vi "ParameterAnalyzer Loop.vi"(6 "Used functions":bool, 8 "error in":errorcluster, 9 "IBM OptoElectroMechanics Configuration":T1={"Parameter Analizer"={"Parameter Analyzer VISA Session"="COM1", "Sweeping Time Parameters"={"Integration Time"=0, "Short Integration Time (s)"=1.0, "Long Integration Time (s)"=0.0, "Wait Time Parameter"=1.0}, "Acquisition Mode"=enum."Sweeping Mode", "Status Polling Time (ms)"=0, "Comment"="Test VI", "SMU 1 - Sweeping"={"Start / Offset"=0.0, "Stop / Ratio"=1.0, "Step \n(linear only)"=0.01, "Compliance"=0.1, "Power \nCompliance"=0.0, "Mode"=0, "Function"=0, "Sweep Mode"=FALSE}, "SMU 2 - Sweeping"={"Start / Offset"=0.0, "Stop / Ratio"=1.0, "Step \n(linear only)"=0.01, "Compliance"=0.1, "Power \nCompliance"=0.0, "Mode"=0, "Function"=0, "Sweep Mode"=FALSE}, "SMU 3 - Sweeping"={"Start / Offset"=0.0, "Stop / Ratio"=1.0, "Step \n(linear only)"=0.01, "Compliance"=0.1, "Power \nCompliance"=0.0, "Mode"=0, "Function"=0, "Sweep Mode"=FALSE}, "SMU 4 - Sweeping"={"Start / Offset"=0.0, "Stop / Ratio"=1.0, "Step \n(linear only)"=0.01, "Compliance"=0.1, "Power \nCompliance"=0.0, "Mode"=0, "Function"=0, "Sweep Mode"=FALSE}, "Sweep Spacing"=0, "Range"=0, "SMU1 - Sampling"={"Source"=10.0, "Compliance"=1e-05, "Mode"=0, "Function"=FALSE}, "SMU2 - Sampling"={"Source"=1.0, "Compliance"=1.0, "Mode"=0, "Function"=FALSE}, "SMU3 - Sampling"={"Source"=10.0, "Compliance"=1e-05, "Mode"=0, "Function"=FALSE}, "SMU4 - Sampling"={"Source"=0.1, "Compliance"=60.0, "Mode"=10, "Function"=FALSE}, "Sampling Time Parameters"={"Initial Interval (s)"=0.1, "Number of Samples"=60, "Total Sampling Time (s)"=10.0, "Hold Time (s)"=0.0, "Sampling Mode"=0, "Sampling Time"=0}, "Stop Condition"={"Enable Delay (s)"=0.0, "Name"="", "Threshold"=0.0, "num. of events"=1, "Event"=0, "Stop Condition Enable"=FALSE}}, "Switching Matrix"={"Switching Matrix VISA Session"="GPIB0::18::INSTR", "Connections"=[{"Connections"=[FALSE, FALSE, FALSE, FALSE, FALSE, FALSE, FALSE, FALSE, FALSE, FALSE, FALSE, FALSE], "Connection Type"=enum."Disconnected"}, {"Connections"=[FALSE, FALSE, FALSE, FALSE, FALSE, FALSE, FALSE, FALSE, FALSE, FALSE, FALSE, FALSE], "Connection Type"=enum."Disconnected"}, {"Connections"=[FALSE, FALSE, FALSE, FALSE, FALSE, FALSE, FALSE, FALSE, FALSE, FALSE, FALSE, FALSE], "Connection Type"=enum."Disconnected"}, {"Connections"=[FALSE, FALSE, FALSE, FALSE, FALSE, FALSE, FALSE, FALSE, FALSE, FALSE, FALSE, FALSE], "Connection Type"=enum."Disconnected"}, {"Connections"=[FALSE, FALSE, FALSE, FALSE, FALSE, FALSE, FALSE, FALSE, FALSE, FALSE, FALSE, FALSE], "Connection Type"=enum."Disconnected"}, {"Connections"=[FALSE, FALSE, FALSE, FALSE, FALSE, FALSE, FALSE, FALSE, FALSE, FALSE, FALSE, FALSE], "Connection Type"=enum."Disconnected"}, {"Connections"=[FALSE, FALSE, FALSE, FALSE, FALSE, FALSE, FALSE, FALSE, FALSE, FALSE, FALSE, FALSE], "Connection Type"=enum."Disconnected"}, {"Connections"=[FALSE, FALSE, FALSE, FALSE, FALSE, FALSE, FALSE, FALSE, FALSE, FALSE, FALSE, FALSE], "Connection Type"=enum."Disconnected"}]}, "Stress Control"={"Stress Control VISA Session"="StrainMotor", "Axis"=0, "Motion"=0, "Destination (°)"=0.0, "Speed (°/s)"=4.0, "Position (°)"=25.0}, "Optical Spectrometer"={"Laser Settings"={"Laser Wavelength"=enum."365 nm", "Neutral Density Filter"=enum."100%"}, "Spectrometer Settings"={"Confocal Hole Size (µm)"=0.0, "Grating"=2, "Detector"=enum."InGaAs Array"}, "Acquisition Settings"={"Acquisition Mode"=enum."Multi-Window", "Spectal Position (nm)"=632.0, "From (nm)"=735.0, "To (nm)"=0.0, "Integration Time (s)"=0.0, "Number of Accumulations"=3, "AutoScanning"=FALSE, "Spike Removal"=FALSE}, "Path"=path "C:/07 - Prizes and Awards/Marie Curie Prize/Reply Editors Final NCOMMS(10).docx"}, "Switches & Mirrors"={"Relay VISA Session"="COM1", "Switches"={"Laser"=FALSE, "Video"=FALSE}, "Delays (ms)"={"Laser"=500, "Video"=1500}}, "Camera"={"Settings"={"Pixel clock"=20, "Frame rate"=30.0, "Exposure time"=33.21525, "Master Gain"=0, "Red Gain"=0, "Green Gain"=0, "Blue Gain"=0, "Auto Gain"=FALSE, "White-balance"=FALSE, "Color Correction"=FALSE}}, "XYZ Stage"={"Connection Settings"={"Tango VISA"="", "Baudrate"=57600, "Show Protocol?"=FALSE}, "Manual Control"={"North"=FALSE, "South"=FALSE, "West"=FALSE, "East"=FALSE, "Up"=FALSE, "Down"=FALSE, "Stop"=FALSE, "XY Step"=0.0, "Z step"=0.0}, "Coordinate Control"={"Motion Mode"=enum."Absolute", "Destination [mm]"=[]}}, "AutoFocus"={"Matching Criteria"={"Minimum Score"=700.0, "Color Score Weight"=700.0, "Minimum Contrast"=50, "Match Mode"=0, "Match Feature Mode"=0, "Subpixel Accuracy"=TRUE, "Color Sensitivity"=1, "Search Strategy"=1}, "Z Scan Parameters"={"Z Range"=1380.0, "Resolution"=5000.0, "Initial Direction"=enum."Up", "Focus Threshold"=0.1, "Ascent Constant"=0.1}, "Displacement"=0.0, "Transformation Matrix"=[]}, "Sava Data"={"Workspace Info"={"Device Name"="ProberHead_Tst_C29K3_7(2)", "Device Info"="ProberHead_Tst_C29", "Path"=path "C:/Users/gio/Desktop/ProbeHeadTest"}, "Instrument Configuration"={"Instrument"=enum."Unknown Instrument", "Configuration"="Test Configuration"}, "Stress Motor Position"=0.0, "Electrical Measurement"={"Sequence"=[], "V1"=[], "V2"=[], "V3"=[], "V4"=[], "I1"=[], "I2"=[], "I3"=[], "I4"=[]}, "Optical Spectrum"={"Intensity"=[], "Wavelength"=[], "Energy"=[], "Raman Shift"=[], "Detector Temperature"=0.0}}, "PlotData"={"Sliders"={"Strain Sequence"=0, "Instrument Sequence"=0}, "Measurement"={"Which Instrument?"=enum."No Plot", "Electrical Measurement"={"Sequence"=[], "V1"=[], "V2"=[], "V3"=[], "V4"=[], "I1"=[], "I2"=[], "I3"=[], "I4"=[]}, "Measurement Mode"=enum."Sweeping Mode", "Optical Spectrum"={"Intensity"=[], "Wavelength"=[], "Energy"=[], "Raman Shift"=[], "Detector Temperature"=0.0}}, "Instrument Steps"=[], "Strain Points"=[]}, "Instrument Sequence"={"Caller VI"=enum."User"}, "Strain Measurement"={"Stress Sequence "={"Max Motor Position"=1380.0, "# Intermediate Points"=5000, "Initial Direction"=enum."Tension"}, "Track?"=FALSE}} {"AutoFocus"."Displacement" scale=1.0..1000.0; "AutoFocus"."Z Scan Parameters"."Focus Threshold" min=0.0 max=1000.0 step=1.0 format="%#_2f"; "AutoFocus"."Z Scan Parameters"."Ascent Constant" min=0.0 max=1000.0 step=1.0 format="%#_2f"; "AutoFocus"."Z Scan Parameters"."Resolution" min=0.0 max=1.0 step=0.01 format="%_2g"; "AutoFocus"."Z Scan Parameters"."Z Range" format="%_3g"; "AutoFocus"."Matching Criteria"."Match Mode" items=["Shift Invariant", "Rotation Invariant"]; "AutoFocus"."Matching Criteria"."Match Feature Mode" items=["Color and Shape", "Color", "Shape"]; "AutoFocus"."Matching Criteria"."Color Sensitivity" items=["Low Sensitivity", "Medium Sensitivity", "High Sensitivity"]; "AutoFocus"."Matching Criteria"."Search Strategy" items=["Conservative", "Balance", "Aggressive", "Very Aggressive"]; "XYZ Stage"."Manual Control"."Z step" scale=0.1..10.0; "XYZ Stage"."Manual Control"."XY Step" scale=0.1..1000.0; "Camera"."Settings"."Blue Gain" min=0 max=100 scale=0.0..100.0; "Camera"."Settings"."Green Gain" min=0 max=100 scale=0.0..100.0; "Camera"."Settings"."Red Gain" min=0 max=100 scale=0.0..100.0; "Camera"."Settings"."Master Gain" min=0 max=100 scale=0.0..100.0; "Camera"."Settings"."Exposure time" min=0.101625 max=159.246375 step=0.101625 scale=0.101625..159.246375 scale format="%#.3g"; "Camera"."Settings"."Frame rate" min=2.7455631699174137 max=6.2675785993528725 step=0.000101625 scale=2.7455631699174137..6.2675785993528725 scale format="%^#_3g"; "Camera"."Settings"."Pixel clock" min=5 max=43 scale=5.0..43.0; "PlotData"."Sliders"."Instrument Sequence" scale=0.0..10.0; "PlotData"."Sliders"."Strain Sequence" scale=0.0..10.0; "Strain Measurement"."Stress Sequence"."# Intermediate Points" max=1390; "Parameter Analizer"."Stop Condition"."Event" items=["Value > Threshold", "Value < Threshold", "| Value | > | Threshold |", "| Value | < | Threshold |"]; "Parameter Analizer"."Stop Condition"."Threshold" format="%^.2e"; "Parameter Analizer"."Stop Condition"."Enable Delay (s)" format="%.1f"; "Parameter Analizer"."Sampling Time Parameters"."Sampling Time" items=["Auto (linear only)", "No Limit", "Set Limit"]; "Parameter Analizer"."Sampling Time Parameters"."Sampling Mode" items=["Linear", "Log10", "Log25", "Log50", "Thinned Out"]; "Parameter Analizer"."Sampling Time Parameters"."Hold Time (s)" format="%.4f"; "Parameter Analizer"."Sampling Time Parameters"."Total Sampling Time (s)" format="%.1f"; "Parameter Analizer"."Sampling Time Parameters"."Initial Interval (s)" format="%^.3e"; "Parameter Analizer"."SMU 4 - Sweeping"."Function" items=["Disabled", "Var 1", "Var 2", "Var 1'", "Constant"]; "Parameter Analizer"."SMU 4 - Sweeping"."Mode" items=["V", "I", "V pulse", "I  pulse", "Common"]; "Parameter Analizer"."SMU 4 - Sweeping"."Power \nCompliance" format="%^.2e"; "Parameter Analizer"."SMU 4 - Sweeping"."Compliance" format="%^.2e"; "Parameter Analizer"."SMU 4 - Sweeping"."Step \n(linear only)" format="%^.4e"; "Parameter Analizer"."SMU 4 - Sweeping"."Stop / Ratio" format="%^.4e"; "Parameter Analizer"."SMU 4 - Sweeping"."Start / Offset" format="%^.4e"; "Parameter Analizer"."SMU 3 - Sweeping"."Function" items=["Disabled", "Var 1", "Var 2", "Var 1'", "Constant"]; "Parameter Analizer"."SMU 3 - Sweeping"."Mode" items=["V", "I", "V pulse", "I  pulse", "Common"]; "Parameter Analizer"."SMU 3 - Sweeping"."Power \nCompliance" format="%^.2e"; "Parameter Analizer"."SMU 3 - Sweeping"."Compliance" format="%^.2e"; "Parameter Analizer"."SMU 3 - Sweeping"."Step \n(linear only)" format="%^.4e"; "Parameter Analizer"."SMU 3 - Sweeping"."Stop / Ratio" format="%^.4e"; "Parameter Analizer"."SMU 3 - Sweeping"."Start / Offset" format="%^.4e"; "Parameter Analizer"."SMU 2 - Sweeping"."Function" items=["Disabled", "Var 1", "Var 2", "Var 1'", "Constant"]; "Parameter Analizer"."SMU 2 - Sweeping"."Mode" items=["V", "I", "V pulse", "I  pulse", "Common"]; "Parameter Analizer"."SMU 2 - Sweeping"."Power \nCompliance" format="%^.2e"; "Parameter Analizer"."SMU 2 - Sweeping"."Compliance" format="%^.2e"; "Parameter Analizer"."SMU 2 - Sweeping"."Step \n(linear only)" format="%^.4e"; "Parameter Analizer"."SMU 2 - Sweeping"."Stop / Ratio" format="%^.4e"; "Parameter Analizer"."SMU 2 - Sweeping"."Start / Offset" format="%^.4e"; "Parameter Analizer"."SMU 1 - Sweeping"."Function" items=["Disabled", "Var 1", "Var 2", "Var 1'", "Constant"]; "Parameter Analizer"."SMU 1 - Sweeping"."Mode" items=["V", "I", "V pulse", "I  pulse", "Common"]; "Parameter Analizer"."SMU 1 - Sweeping"."Power \nCompliance" format="%^.2e"; "Parameter Analizer"."SMU 1 - Sweeping"."Compliance" format="%^.2e"; "Parameter Analizer"."SMU 1 - Sweeping"."Step \n(linear only)" format="%^.4e"; "Parameter Analizer"."SMU 1 - Sweeping"."Stop / Ratio" format="%^.4e"; "Parameter Analizer"."SMU 1 - Sweeping"."Start / Offset" format="%^.4e"; "Parameter Analizer"."Sweeping Time Parameters"."Long Integration Time (s)" scale=0.02..2.0; "Parameter Analizer"."Sweeping Time Parameters"."Short Integration Time (s)" scale=8e-05..0.00192; "Parameter Analizer"."Sweeping Time Parameters"."Integration Time" items=["Short", "Long"]; "Parameter Analizer"."Sweeping Time Parameters"."Wait Time Parameter" format="%.1f"; "Parameter Analizer"."SMU4 - Sampling"."Mode" items=["V", "I", "Common"]; "Parameter Analizer"."SMU4 - Sampling"."Compliance" format="%^.2e"; "Parameter Analizer"."SMU4 - Sampling"."Source" format="%^.3e"; "Parameter Analizer"."SMU3 - Sampling"."Mode" items=["V", "I", "Common"]; "Parameter Analizer"."SMU3 - Sampling"."Compliance" format="%^.2e"; "Parameter Analizer"."SMU3 - Sampling"."Source" format="%^.3e"; "Parameter Analizer"."SMU2 - Sampling"."Mode" items=["V", "I", "Common"]; "Parameter Analizer"."SMU2 - Sampling"."Compliance" format="%^.2e"; "Parameter Analizer"."SMU2 - Sampling"."Source" format="%^.3e"; "Parameter Analizer"."SMU1 - Sampling"."Mode" items=["V", "I", "Common"]; "Parameter Analizer"."SMU1 - Sampling"."Compliance" format="%^.2e"; "Parameter Analizer"."SMU1 - Sampling"."Source" format="%^.3e"; "Parameter Analizer"."Range" items=["auto", "fixed", "limited"]; "Parameter Analizer"."Sweep Spacing" items=["linear", "log 10", "log 25", "log 50"]; "Stress Control"."Axis" min=1 max=3; "Stress Control"."Position (°)" format="%.6g"; "Stress Control"."Speed (°/s)" min=0.0 max=4.0 format="%.6f"; "Stress Control"."Destination (°)" min=-2000000000.0 max=2000000000.0 format="%.6f"; "Stress Control"."Motion" items=["Absolute", "Relative"]; "Optical Spectrometer"."Spectrometer Settings"."Grating" items=["1800 l/mm", "150 l/mm"]}, 10 "Message Queues out":T57, 11 "Notifiers":T44) -> (0 "error out":errorcluster)   [LabVIEW 2014]
uses:
  support/Message Queue/All Message Queues.ctl
  support/Message Queue/Message Cluster.ctl
  support/Notifiers/Notifiers.ctl
  support/Message Handler Loop Notifiers.ctl
  Hardware Control/Parameter Analyzer/Parameter Analyzer Notifiers.ctl
  Hardware Control/Switching Matrix/Switching Matrix Notifiers.ctl
  Hardware Control/Stress Control/StressControl Notifiers.ctl
  Hardware Control/Spectrometer/Spectrometer Notifiers.ctl
  Hardware Control/Switches and Mirrors/SwitchesMirrors Notifiers.ctl
  Hardware Control/Camera/Camera Notifiers.ctl
  Hardware Control/XYZ Stage/XYZ Notifications.ctl
  Hardware Control/Autofocus/Autofocus Notifiers.ctl
  Measurements/Optoelectronic Measurement/Optoelectronic Notifiers.ctl
  Measurements/Save Data/SaveData Notifiers.ctl
  Measurements/Instrument Sequence/Instrument Sequence Notifiers.ctl
  support/Configuration/Configuration.ctl
  Hardware Control/Parameter Analyzer/Parameter Analyzer Config.ctl
  Hardware Control/Parameter Analyzer/Parameter Analyzer Integration Parameters.ctl
  Hardware Control/Parameter Analyzer/Parameter Analyzer SMU Sweeping.ctl
  Hardware Control/Parameter Analyzer/Parameter Analyzer Sweep Spacing.ctl
  Hardware Control/Parameter Analyzer/Parameter Analyzer SMU Range.ctl
  Hardware Control/Parameter Analyzer/Parameter Analyzer SMU Sampling.ctl
  Hardware Control/Parameter Analyzer/Parameter Analyzer Sampling Parameters.ctl
  Hardware Control/Parameter Analyzer/Parameter Analyzer Stop Sampling Conditions.ctl
  Hardware Control/Switching Matrix/Switching Matrix Config.ctl
  Hardware Control/Stress Control/StressControl Config.ctl
  Hardware Control/Spectrometer/Spectrometer Config.ctl
  Hardware Control/Spectrometer/Laser Settings.ctl
  Hardware Control/Spectrometer/Laser.ctl
  Hardware Control/Spectrometer/Filter.ctl
  Hardware Control/Spectrometer/Grating Detector Settings.ctl
  Hardware Control/Spectrometer/Grating.ctl
  Hardware Control/Spectrometer/Detector.ctl
  Hardware Control/Spectrometer/Acquisition Settings.ctl
  Hardware Control/Switches and Mirrors/SwitchesMirrors Config.ctl
  Hardware Control/Switches and Mirrors/SwitchesMirrors Status.ctl
  Hardware Control/Camera/Camera Config.ctl
  Hardware Control/Camera/Camera Settings.ctl
  Hardware Control/XYZ Stage/XYZ Config.ctl
  Hardware Control/XYZ Stage/XYZ Connection Settings.ctl
  Hardware Control/XYZ Stage/XYZ Stage Control.ctl
  Hardware Control/XYZ Stage/XYZ Coordinate Control.ctl
  Hardware Control/Autofocus/AutoFocus Config.ctl
  Hardware Control/Autofocus/ZScan.ctl
  <vilib>/Analysis/Matrix/Datatypes/RealMatrix.ctl
  Measurements/Save Data/SaveData Config.ctl
  Measurements/Save Data/SaveData Workspace Info.ctl
  Measurements/Save Data/SaveData Instrument Configuration.ctl
  Measurements/Instrument Sequence/Instrument List.ctl
  Hardware Control/Spectrometer/Spectral Data.ctl
  Measurements/Plot Data/PlotData Config.ctl
  Measurements/Plot Data/Measurement.ctl
  Measurements/Plot Data/WhichInstrument.ctl
  Hardware Control/Parameter Analyzer/Electrical Data.ctl
  Measurements/Instrument Sequence/Instrument Steps.ctl
  Measurements/Instrument Sequence/Action.ctl
  Measurements/Instrument Sequence/Instrument Sequence Config.ctl
  Measurements/Strain Measurement/Strain Measurement Config.ctl
  Hardware Control/Parameter Analyzer/Parameter Analyzer Functions.ctl
  support/Message Queue/Message Queue.lvlib
  <vilib>/Analysis/Matrix/NI_Matrix.lvlib
panel:
  # "LICENSED MATERIALS – PROPERTY OF IBM\nCopyright IBM Corp. 2016,\nALL RIGHTS RESERVED"
  # "XY"
  # "Z"
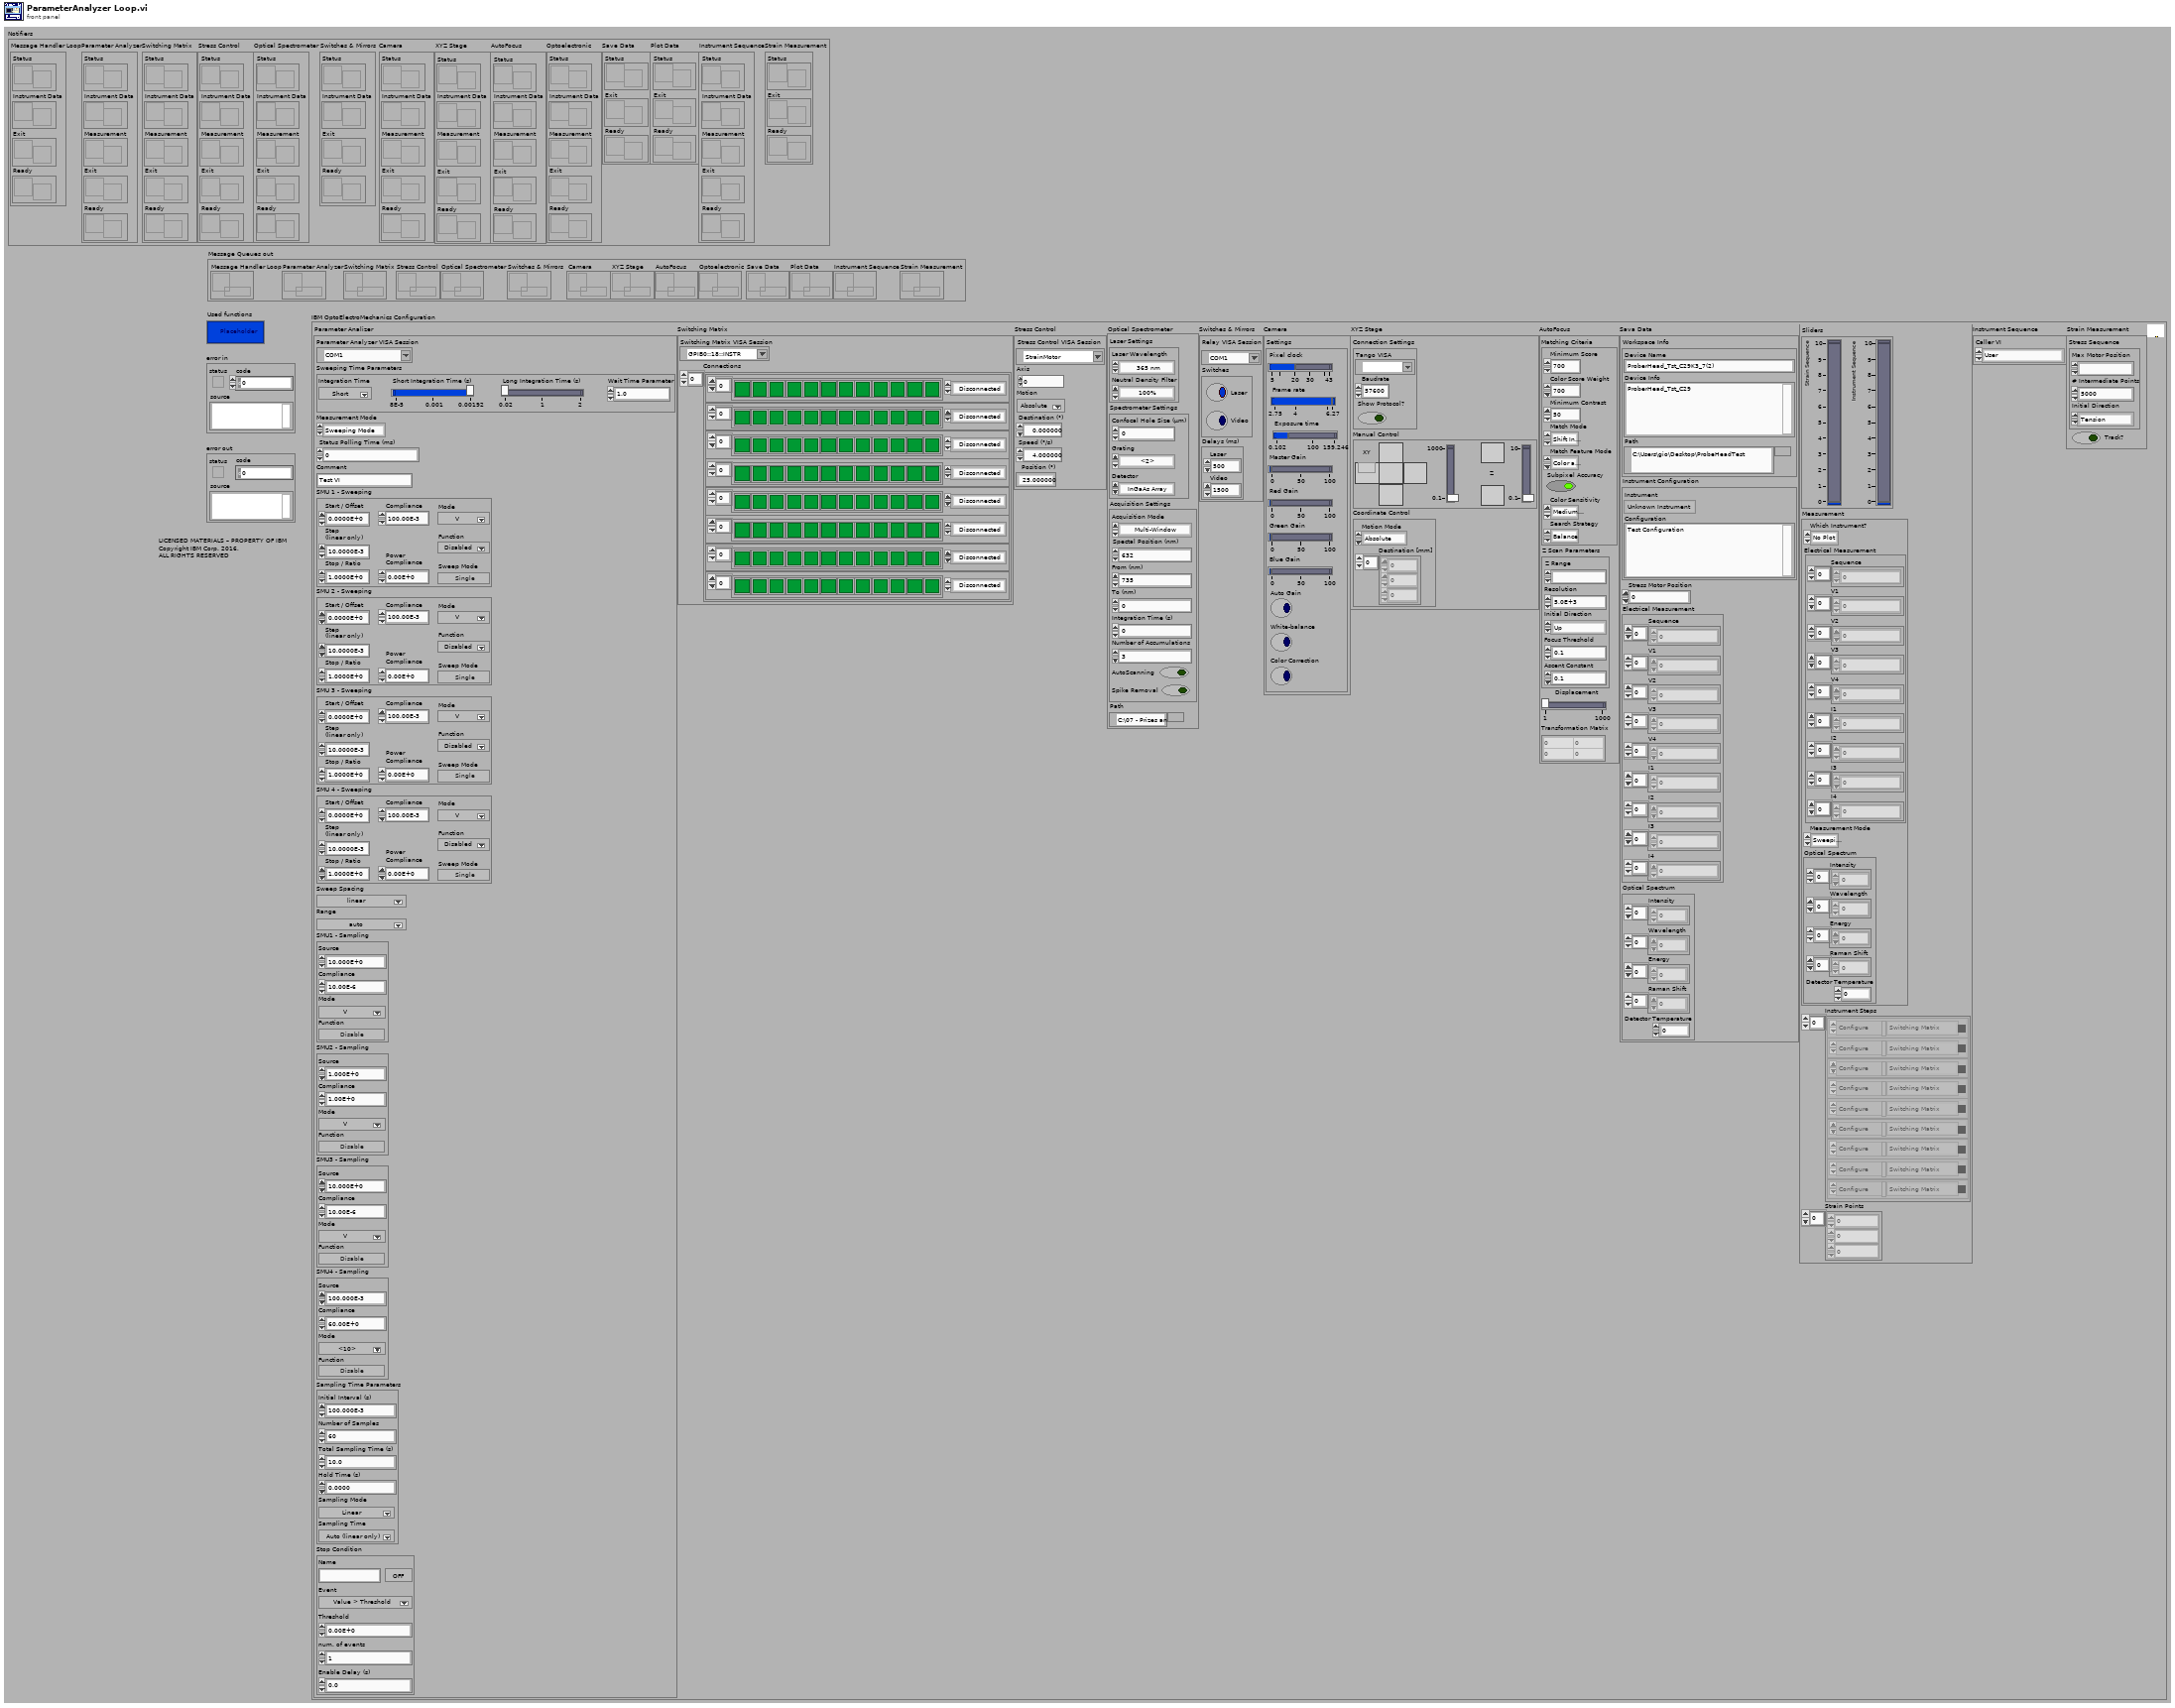
[diagram p1: front panel]
types:
  T1 = typedef "Configuration.ctl" = cluster{"Parameter Analizer":T2, "Switching Matrix":T10, "Stress Control":T11, "Optical Spectrometer":T12, "Switches & Mirrors":T20, "Camera":T22, "XYZ Stage":T24, "AutoFocus":T28, "Sava Data":T31, "PlotData":T36, "Instrument Sequence":T42, "Strain Measurement":T43}
  T2 = typedef "Parameter Analyzer Config.ctl" = cluster{"Parameter Analyzer VISA Session":refnum<visa-resource-name>, "Sweeping Time Parameters":T3, "Acquisition Mode":enum32{"Sweeping Mode", "Sampling Mode"}, "Status Polling Time (ms)":u32, "Comment":string, "SMU 1 - Sweeping":T4, "SMU 2 - Sweeping":T4, "SMU 3 - Sweeping":T4, "SMU 4 - Sweeping":T4, "Sweep Spacing":T5, "Range":T6, "SMU1 - Sampling":T7, "SMU2 - Sampling":T7, "SMU3 - Sampling":T7, "SMU4 - Sampling":T7, "Sampling Time Parameters":T8, "Stop Condition":T9}
  T3 = typedef "Parameter Analyzer Integration Parameters.ctl" = cluster{"Integration Time":u32, "Short Integration Time (s)":dbl, "Long Integration Time (s)":dbl, "Wait Time Parameter":dbl}
  T4 = typedef "Parameter Analyzer SMU Sweeping.ctl" = cluster{"Start / Offset":dbl, "Stop / Ratio":dbl, "Step \n(linear only)":dbl, "Compliance":dbl, "Power \nCompliance":dbl, "Mode":u32, "Function":i32, "Sweep Mode":bool}
  T5 = typedef "Parameter Analyzer Sweep Spacing.ctl" = u16
  T6 = typedef "Parameter Analyzer SMU Range.ctl" = u16
  T7 = typedef "Parameter Analyzer SMU Sampling.ctl" = cluster{"Source":dbl, "Compliance":dbl, "Mode":u32, "Function":bool}
  T8 = typedef "Parameter Analyzer Sampling Parameters.ctl" = cluster{"Initial Interval (s)":dbl, "Number of Samples":i32, "Total Sampling Time (s)":dbl, "Hold Time (s)":dbl, "Sampling Mode":i32, "Sampling Time":i32}
  T9 = typedef "Parameter Analyzer Stop Sampling Conditions.ctl" = cluster{"Enable Delay (s)":dbl, "Name":string, "Threshold":dbl, "num. of events":i32, "Event":i32, "Stop Condition Enable":bool}
  T10 = typedef "Switching Matrix Config.ctl" = cluster{"Switching Matrix VISA Session":refnum<visa-resource-name>, "Connections":cluster{"Connections":bool[], "Connection Type":enum16{"Disconnected", "Make - Break", "Break - Make"}}[]}
  T11 = typedef "StressControl Config.ctl" = cluster{"Stress Control VISA Session":refnum<visa-resource-name>, "Axis":i32, "Motion":u16, "Destination (°)":dbl, "Speed (°/s)":dbl, "Position (°)":dbl}
  T12 = typedef "Spectrometer Config.ctl" = cluster{"Laser Settings":T13, "Spectrometer Settings":T16, "Acquisition Settings":T19, "Path":path}
  T13 = typedef "Laser Settings.ctl" = cluster{"Laser Wavelength":T14, "Neutral Density Filter":T15}
  T14 = typedef "Laser.ctl" = enum16{"633 nm", "784 nm", "532 nm", "365 nm"}
  T15 = typedef "Filter.ctl" = enum16{"100%", "50%", "25%", "10%", "1%", "0.1%", "0.01%"}
  T16 = typedef "Grating Detector Settings.ctl" = cluster{"Confocal Hole Size (µm)":dbl, "Grating":T17, "Detector":T18}
  T17 = typedef "Grating.ctl" = u16
  T18 = typedef "Detector.ctl" = enum16{"InGaAs Array", "Silicon CCD"}
  T19 = typedef "Acquisition Settings.ctl" = cluster{"Acquisition Mode":enum16{"Single Window", "Multi-Window"}, "Spectal Position (nm)":dbl, "From (nm)":dbl, "To (nm)":dbl, "Integration Time (s)":dbl, "Number of Accumulations":i32, "AutoScanning":bool, "Spike Removal":bool}
  T20 = typedef "SwitchesMirrors Config.ctl" = cluster{"Relay VISA Session":refnum<visa-resource-name>, "Switches":T21, "Delays (ms)":cluster{"Laser":u32, "Video":u32}}
  T21 = typedef "SwitchesMirrors Status.ctl" = cluster{"Laser":bool, "Video":bool}
  T22 = typedef "Camera Config.ctl" = cluster{"Settings":T23}
  T23 = typedef "Camera Settings.ctl" = cluster{"Pixel clock":i32, "Frame rate":dbl, "Exposure time":dbl, "Master Gain":i32, "Red Gain":i32, "Green Gain":i32, "Blue Gain":i32, "Auto Gain":bool, "White-balance":bool, "Color Correction":bool}
  T24 = typedef "XYZ Config.ctl" = cluster{"Connection Settings":T25, "Manual Control":T26, "Coordinate Control":T27}
  T25 = typedef "XYZ Connection Settings.ctl" = cluster{"Tango VISA":refnum<visa-resource-name>, "Baudrate":i32, "Show Protocol?":bool}
  T26 = typedef "XYZ Stage Control.ctl" = cluster{"North":bool, "South":bool, "West":bool, "East":bool, "Up":bool, "Down":bool, "Stop":bool, "XY Step":dbl, "Z step":dbl}
  T27 = typedef "XYZ Coordinate Control.ctl" = cluster{"Motion Mode":enum16{"Absolute", "Relative"}, "Destination [mm]":dbl[]}
  T28 = typedef "AutoFocus Config.ctl" = cluster{"Matching Criteria":cluster{"Minimum Score":sgl, "Color Score Weight":sgl, "Minimum Contrast":i32, "Match Mode":u32, "Match Feature Mode":u32, "Subpixel Accuracy":bool, "Color Sensitivity":u32, "Search Strategy":u32}, "Z Scan Parameters":T29, "Displacement":dbl, "Transformation Matrix":T30}
  T29 = typedef "ZScan.ctl" = cluster{"Z Range":ext, "Resolution":dbl, "Initial Direction":enum16{"Up", "Down"}, "Focus Threshold":dbl, "Ascent Constant":dbl}
  T30 = typedef "NI_Matrix.lvlib/RealMatrix.ctl" = dbl[][]
  T31 = typedef "SaveData Config.ctl" = cluster{"Workspace Info":T32, "Instrument Configuration":T33, "Stress Motor Position":dbl, "Electrical Measurement":cluster{"Sequence":dbl[], "V1":dbl[], "V2":dbl[], "V3":dbl[], "V4":dbl[], "I1":dbl[], "I2":dbl[], "I3":dbl[], "I4":dbl[]}, "Optical Spectrum":T35}
  T32 = typedef "SaveData Workspace Info.ctl" = cluster{"Device Name":string, "Device Info":string, "Path":path}
  T33 = typedef "SaveData Instrument Configuration.ctl" = cluster{"Instrument":T34, "Configuration":string}
  T34 = typedef "Instrument List.ctl" = enum32{"Unknown Instrument", "Switching Matrix", "Parameter Analyzer", "Optical Spectrometer", "Optoelectronic", "Autofocus"}
  T35 = typedef "Spectral Data.ctl" = cluster{"Intensity":dbl[], "Wavelength":dbl[], "Energy":dbl[], "Raman Shift":dbl[], "Detector Temperature":dbl}
  T36 = typedef "PlotData Config.ctl" = cluster{"Sliders":cluster{"Strain Sequence":i32, "Instrument Sequence":i32}, "Measurement":T37, "Instrument Steps":T40, "Strain Points":dbl[]}
  T37 = typedef "Measurement.ctl" = cluster{"Which Instrument?":T38, "Electrical Measurement":T39, "Measurement Mode":enum16{"Sweeping Mode", "Sampling Mode"}, "Optical Spectrum":T35}
  T38 = typedef "WhichInstrument.ctl" = enum16{"No Plot", "Spectrometer", "Parameter Analyzer", "Optoelectronic"}
  T39 = typedef "Electrical Data.ctl" = cluster{"Sequence":dbl[], "V1":dbl[], "V2":dbl[], "V3":dbl[], "V4":dbl[], "I1":dbl[], "I2":dbl[], "I3":dbl[], "I4":dbl[]}
  T40 = typedef "Instrument Steps.ctl" = cluster{"Action":T41, "Configuration":variant, "Instrument":T34, "Status":enum8{"False", "True", "Mixed"}}[]
  T41 = typedef "Action.ctl" = enum32{"Configure", "Measure"}
  T42 = typedef "Instrument Sequence Config.ctl" = cluster{"Caller VI":enum16{"User", "Stress Measurement VI"}}
  T43 = typedef "Strain Measurement Config.ctl" = cluster{"Stress Sequence ":cluster{"Max Motor Position":ext, "# Intermediate Points":u32, "Initial Direction":enum16{"Tension", "Compression"}}, "Track?":bool}
  T44 = typedef "Notifiers.ctl" = cluster{"Message Handler Loop":T45, "Parameter Analyzer":T46, "Switching Matrix":T47, "Stress Control":T48, "Optical Spectrometer":T49, "Switches & Mirrors":T50, "Camera":T51, "XYZ Stage":T52, "AutoFocus":T53, "Optoelectronic":T54, "Save Data":T55, "Plot Data":T55, "Instrument Sequence":T56, "Strain Measurement":cluster{"Status":refnum<notifier>, "Exit":refnum<notifier>, "Ready":refnum<notifier>}}
  T45 = typedef "Message Handler Loop Notifiers.ctl" = cluster{"Status":refnum<notifier>, "Instrument Data":refnum<notifier>, "Exit":refnum<notifier>, "Ready":refnum<notifier>}
  T46 = typedef "Parameter Analyzer Notifiers.ctl" = cluster{"Status":refnum<notifier>, "Instrument Data":refnum<notifier>, "Measurement":refnum<notifier>, "Exit":refnum<notifier>, "Ready":refnum<notifier>}
  T47 = typedef "Switching Matrix Notifiers.ctl" = cluster{"Status":refnum<notifier>, "Instrument Data":refnum<notifier>, "Measurement":refnum<notifier>, "Exit":refnum<notifier>, "Ready":refnum<notifier>}
  T48 = typedef "StressControl Notifiers.ctl" = cluster{"Status":refnum<notifier>, "Instrument Data":refnum<notifier>, "Measurement":refnum<notifier>, "Exit":refnum<notifier>, "Ready":refnum<notifier>}
  T49 = typedef "Spectrometer Notifiers.ctl" = cluster{"Status":refnum<notifier>, "Instrument Data":refnum<notifier>, "Measurement":refnum<notifier>, "Exit":refnum<notifier>, "Ready":refnum<notifier>}
  T50 = typedef "SwitchesMirrors Notifiers.ctl" = cluster{"Status":refnum<notifier>, "Instrument Data":refnum<notifier>, "Exit":refnum<notifier>, "Ready":refnum<notifier>}
  T51 = typedef "Camera Notifiers.ctl" = cluster{"Status":refnum<notifier>, "Instrument Data":refnum<notifier>, "Measurement":refnum<notifier>, "Exit":refnum<notifier>, "Ready":refnum<notifier>}
  T52 = typedef "XYZ Notifications.ctl" = cluster{"Status":refnum<notifier>, "Instrument Data":refnum<notifier>, "Measurement":refnum<notifier>, "Exit":refnum<notifier>, "Ready":refnum<notifier>}
  T53 = typedef "Autofocus Notifiers.ctl" = cluster{"Status":refnum<notifier>, "Instrument Data":refnum<notifier>, "Measurement":refnum<notifier>, "Exit":refnum<notifier>, "Ready":refnum<notifier>}
  T54 = typedef "Optoelectronic Notifiers.ctl" = cluster{"Status":refnum<notifier>, "Instrument Data":refnum<notifier>, "Measurement":refnum<notifier>, "Exit":refnum<notifier>, "Ready":refnum<notifier>}
  T55 = typedef "SaveData Notifiers.ctl" = cluster{"Status":refnum<notifier>, "Exit":refnum<notifier>, "Ready":refnum<notifier>}
  T56 = typedef "Instrument Sequence Notifiers.ctl" = cluster{"Status":refnum<notifier>, "Instrument Data":refnum<notifier>, "Measurement":refnum<notifier>, "Exit":refnum<notifier>, "Ready":refnum<notifier>}
  T57 = typedef "Message Queue.lvlib/All Message Queues.ctl" = cluster{"Message Handler Loop":refnum<queue>, "Parameter Analyzer":refnum<queue>, "Switching Matrix":refnum<queue>, "Stress Control":refnum<queue>, "Optical Spectrometer":refnum<queue>, "Switches & Mirrors":refnum<queue>, "Camera":refnum<queue>, "XYZ Stage":refnum<queue>, "AutoFocus":refnum<queue>, "Optoelectronic":refnum<queue>, "Save Data":refnum<queue>, "Plot Data":refnum<queue>, "Instrument Sequence":refnum<queue>, "Strain Measurement":refnum<queue>}
  T58 = typedef "Parameter Analyzer Data.ctl" = cluster{"Configuration":T2, "Refnums":T59, "Initialization":T61}
  T59 = typedef "Parameter Analyzer Refnums.ctl" = cluster{"Status":refnum<vi>, "Electrical Measurement":refnum<vi>, "Plots":T60, "HP Integration Time":refnum<vi>, "VISA":refnum<vi>, "Sweeping Time Parameters":refnum<vi>, "Acquisition Mode":refnum<vi>, "SMU 1 - Sweeping":refnum<vi>, "SMU 2 - Sweeping":refnum<vi>, "SMU 3 - Sweeping":refnum<vi>, "SMU 4 - Sweeping":refnum<vi>, "Sweep Spacing":refnum<vi>, "Range":refnum<vi>, "SMU1 - Sampling":refnum<vi>, "SMU2 - Sampling":refnum<vi>, "SMU3 - Sampling":refnum<vi>, "SMU4 - Sampling":refnum<vi>, "Sampling Time Parameters":refnum<vi>, "Stop Condition":refnum<vi>, "Instrument Status":refnum<vi>}
  T60 = typedef "Electrical Data Plot Refnums.ctl" = cluster{"Plot List":refnum<vi>, "Voltage Plot":refnum<vi>, "Current Plot":refnum<vi>, "IV Characteristic":refnum<vi>, "dI/dV-V Characteristic":refnum<vi>}
  T61 = typedef "Parameter Analyzer Initialization.ctl" = cluster{"Update Visa Session":bool, "Configure Integration Time":bool, "Configure Acquisition Mode":bool, "Update Refnums":bool}
  T62 = typedef "Parameter Analyzer Functions.ctl" = enum16{"Connect", "Configure Sweeping", "Configure Sampling", "Configure Integration Time", "Measure", "Error Check", "Disconnect", "Update Refnums"}
  T63 = cluster{"Sequence":dbl[], "V1":dbl[], "V2":dbl[], "V3":dbl[], "V4":dbl[], "I1":dbl[], "I2":dbl[], "I3":dbl[], "I4":dbl[]}
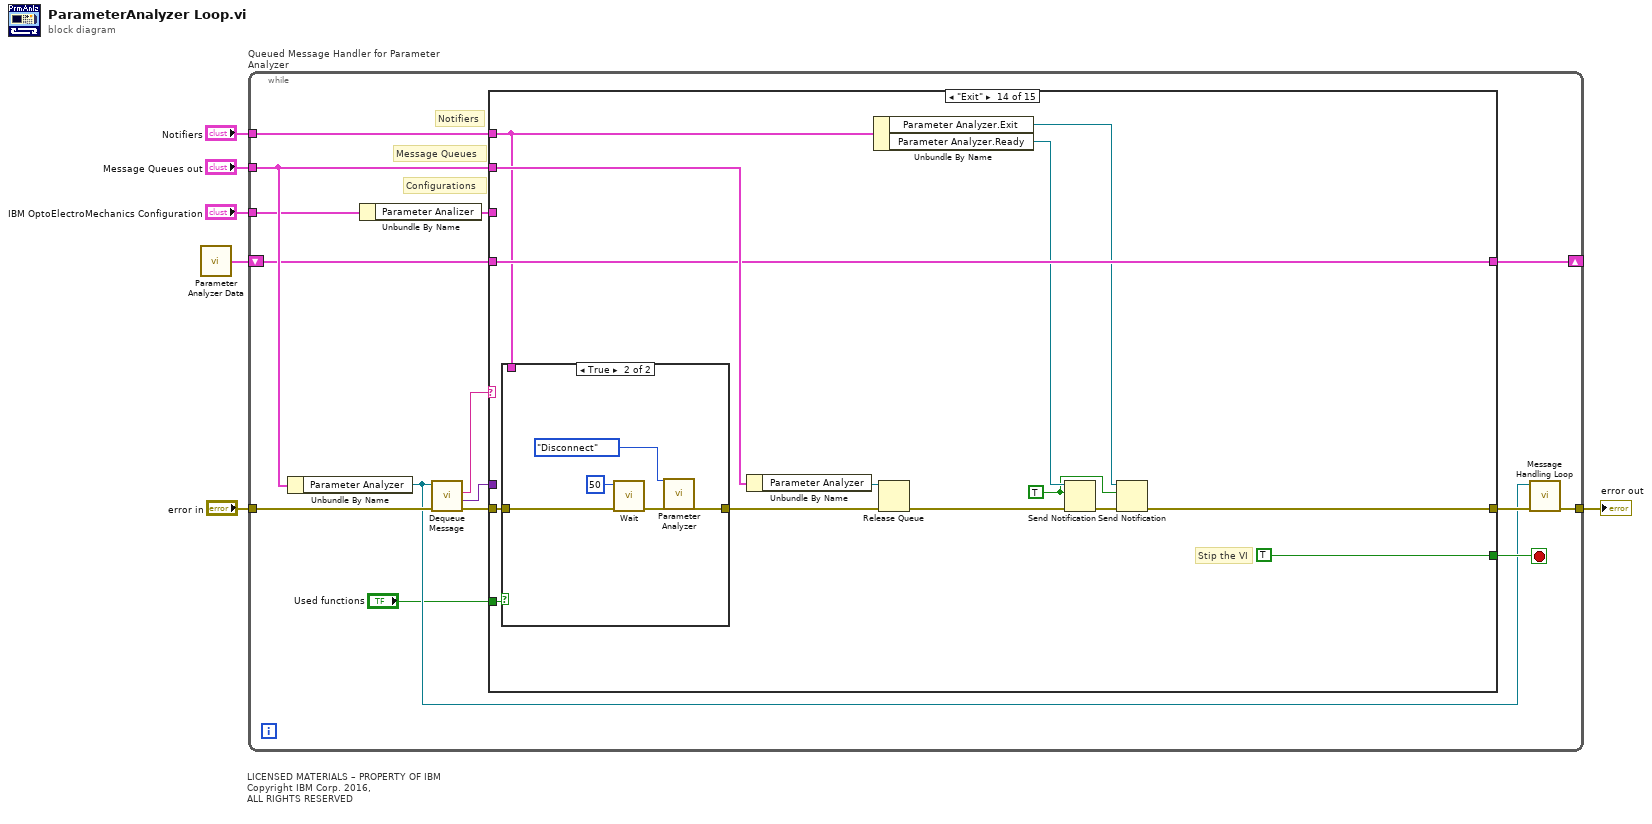
[diagram p0: block diagram]
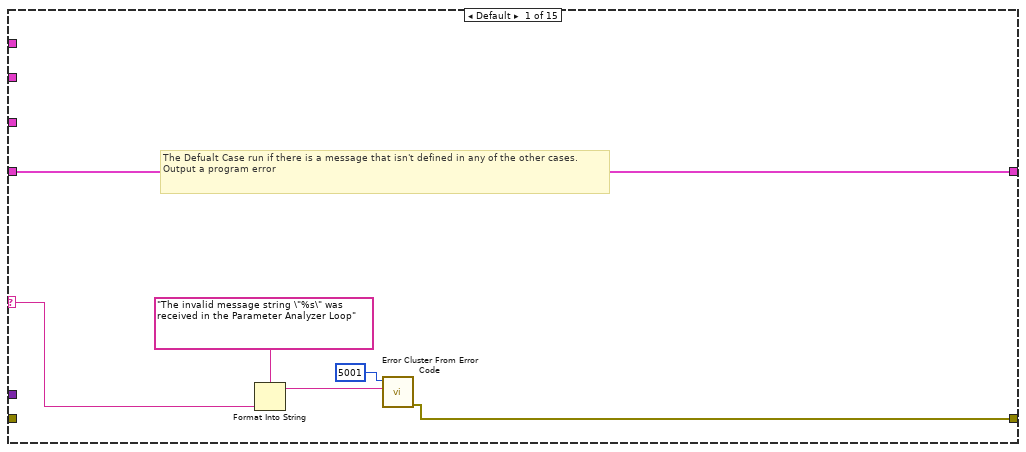
[diagram p2: hidden frame]
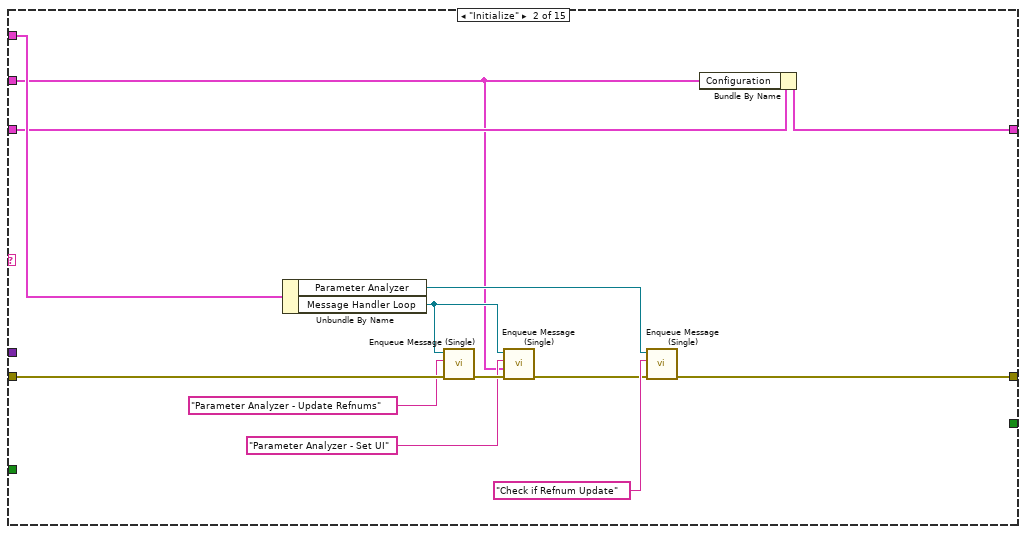
[diagram p3: hidden frame]
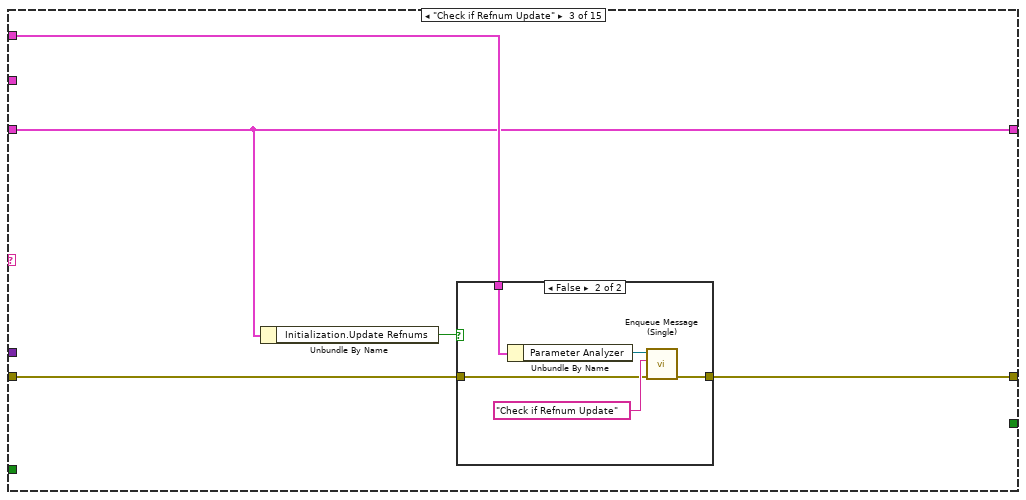
[diagram p4: hidden frame]
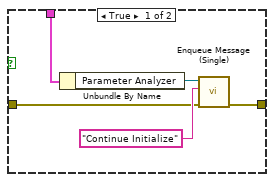
[diagram p5: hidden frame]
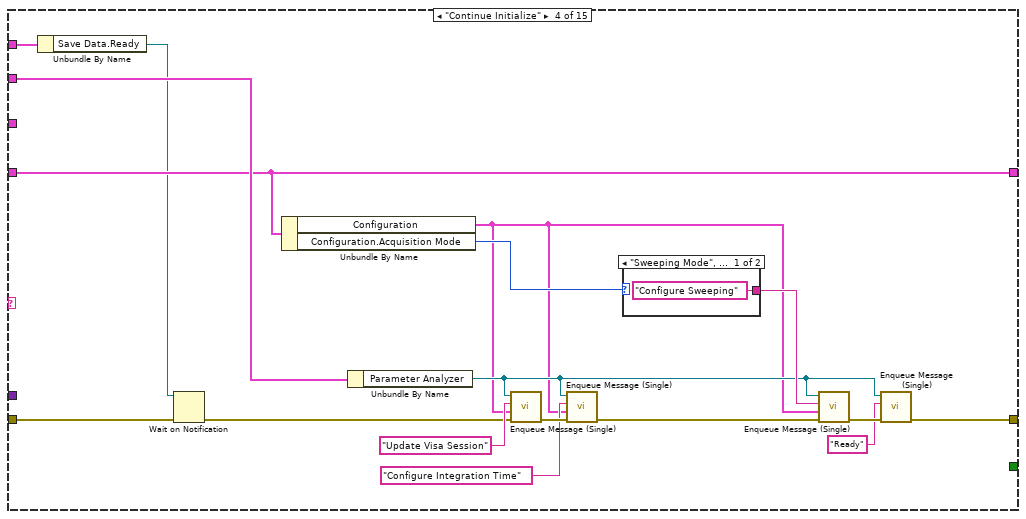
[diagram p6: hidden frame]
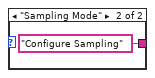
[diagram p7: hidden frame]
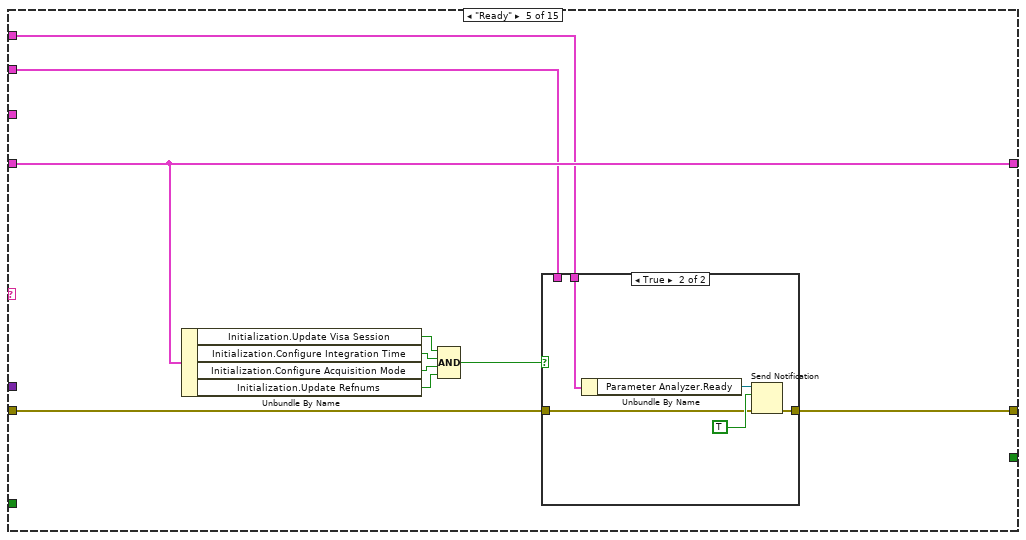
[diagram p8: hidden frame]
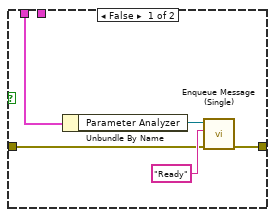
[diagram p9: hidden frame]
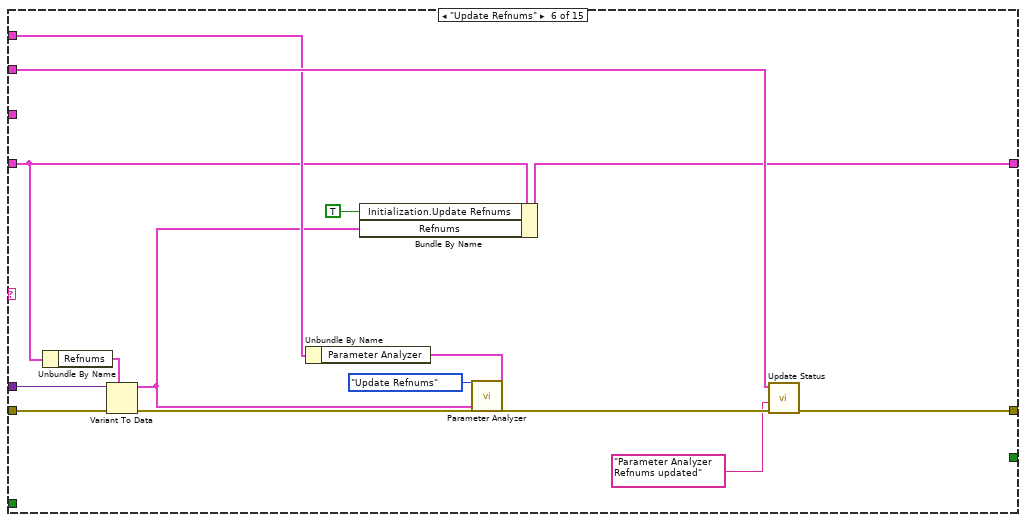
[diagram p10: hidden frame]
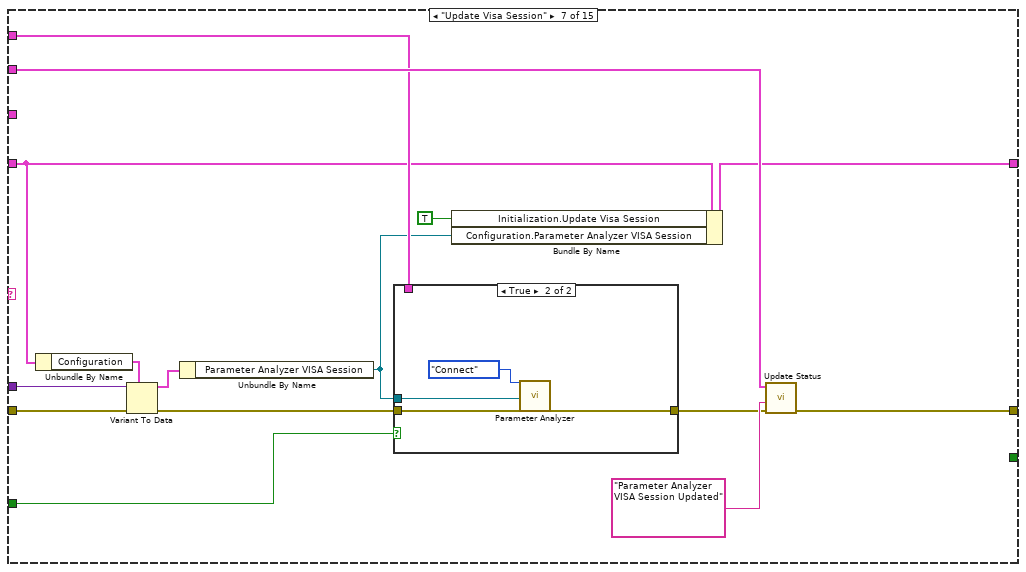
[diagram p11: hidden frame]
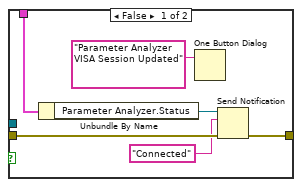
[diagram p12: hidden frame]
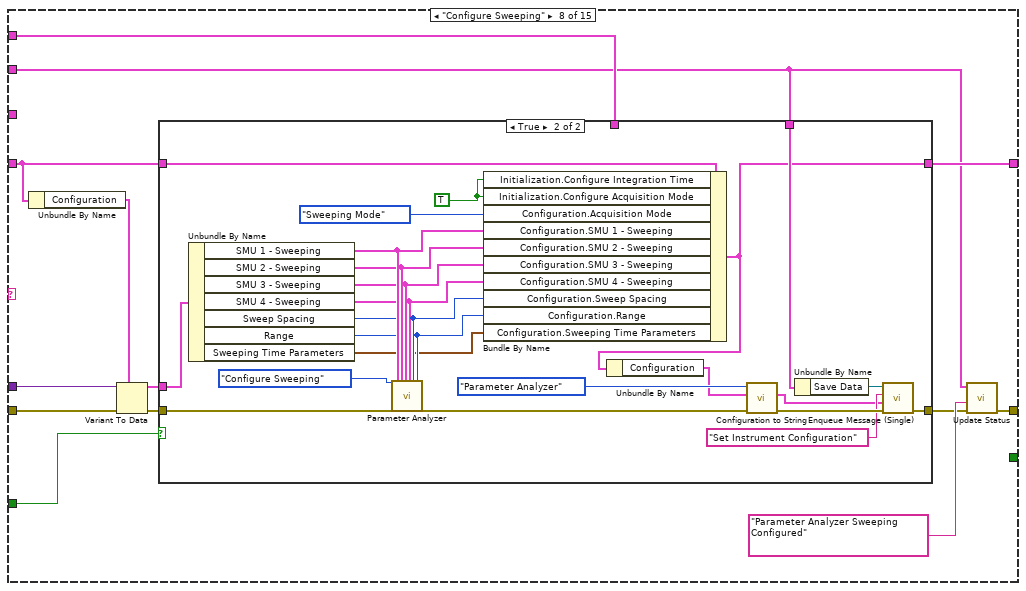
[diagram p13: hidden frame]
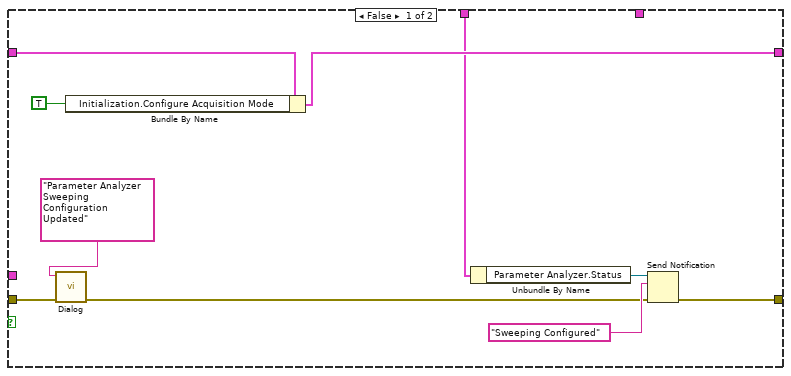
[diagram p14: hidden frame]
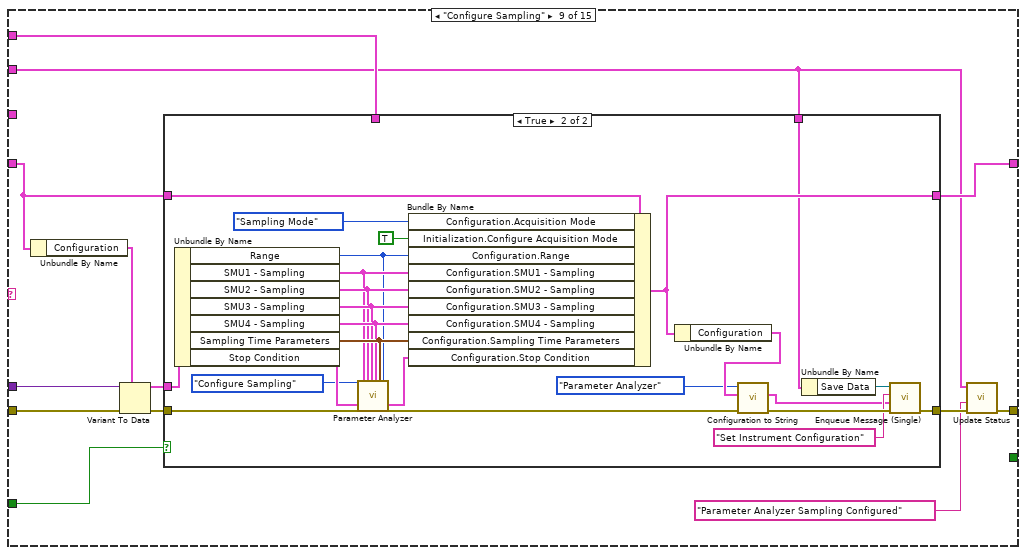
[diagram p15: hidden frame]
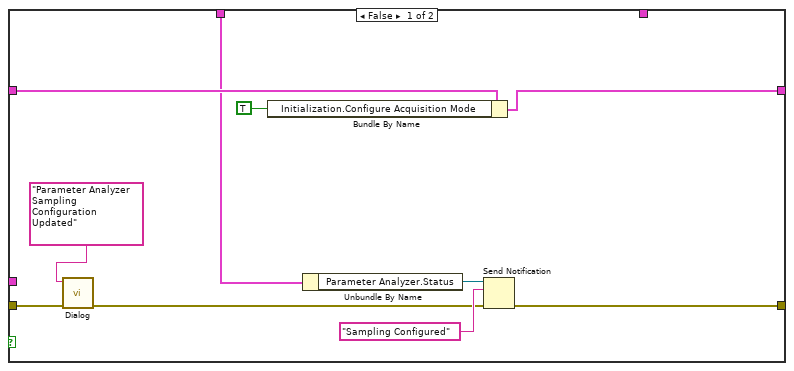
[diagram p16: hidden frame]
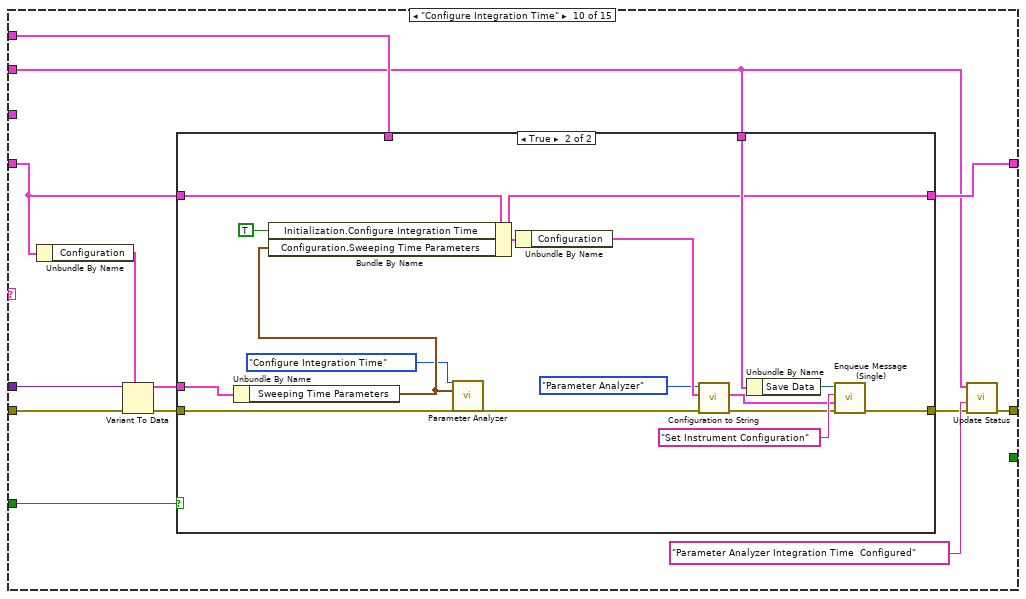
[diagram p17: hidden frame]
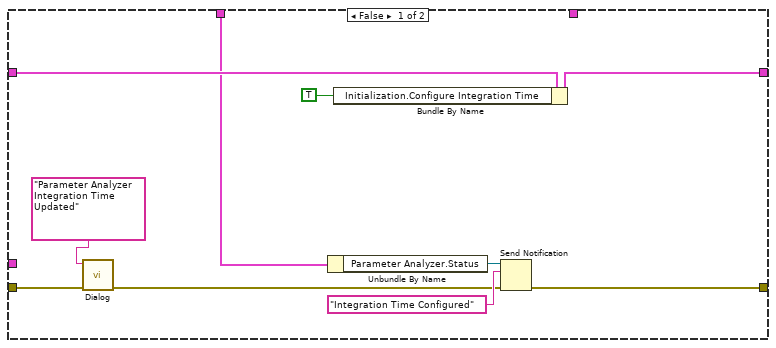
[diagram p18: hidden frame]
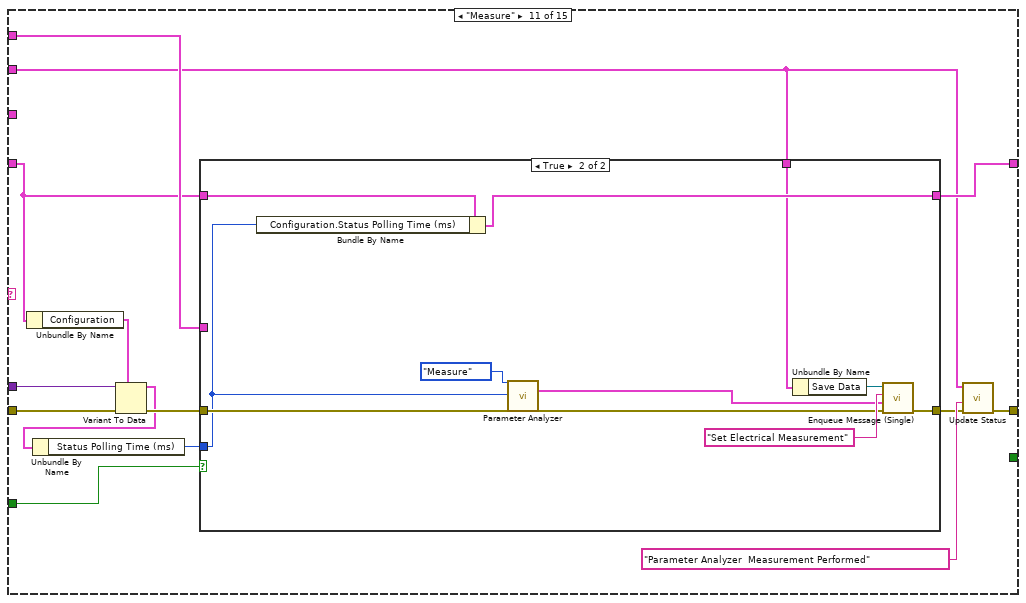
[diagram p19: hidden frame]
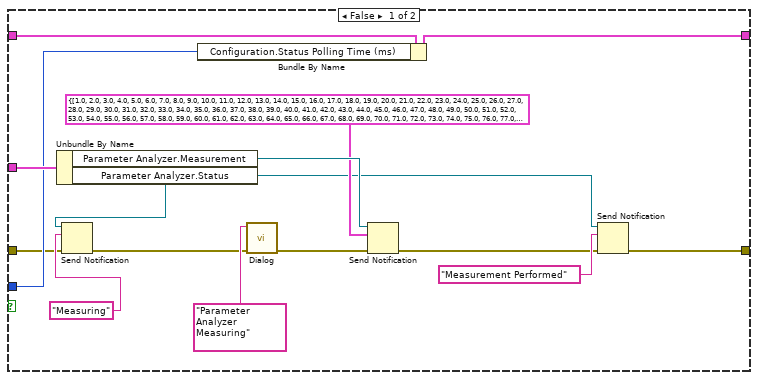
[diagram p20: hidden frame]
diagram:
  # "LICENSED MATERIALS – PROPERTY OF IBM\nCopyright IBM Corp. 2016,\nALL RIGHTS RESERVED"
  n1 = call "Parameter Analyzer Data.vi"() -> ("HP4155C Data"=w1:T58)
  n2 = while "Queued Message Handler for Parameter Analyzer" {
    tunnel: "error in" -> [w21]
    tunnel: [w13] -> w2
    tunnel: "Message Queues out" -> [w17]
    tunnel: "Notifiers" -> [w16]
    tunnel: "IBM OptoElectroMechanics Configuration" -> [w11]
    shift-right: [w7] -> _
    shift-left: w1 -> [w8]
    stop <- w15 stop-if-true
    # "Configurations"
    # "Notifiers"
    # "Message Queues"
    n3 = Unbundle By Name(w17) -> ("Parameter Analyzer"=w12:refnum<queue>)
    n4 = Unbundle By Name(w11) -> ("Parameter Analizer"=w10:T2)
    n5 = call "Dequeue Message.vi"("error in (no error)"=w21, "Message Queue"=w12) -> ("error out"=w20:errorcluster, "Message Data"=w18:variant, "Message"=w19:string)  [unwired: 7 out]
    n6 = case shown="\"Exit\"" w19 {
      selector: w19 -> [w24 _ _ _ _ _ _ _ _ _ _ _ _ _ _]
      tunnel: w20 -> [_ w36 w43 w57 w78 w107 w122 w145 w191 w236 w273 w310 w328 w346 w364]
      tunnel: [w23 w28 w44 w65 w76 w106 w120 w143 w189 w234 w276 w309 w323 w336 w363] -> w14
      tunnel: w18 -> [_ _ _ _ _ w109 w124 w147 w193 w238 w266 _ w321 _ _]
      tunnel: w17 -> [_ w40 w45 w71 w77 w103 w119 w135 w181 w226 w265 w311 w329 w348 _]
      tunnel: w16 -> [_ _ _ w58 w75 w102 w115 w136 w182 w227 w274 _ _ w338 w362]
      tunnel: [_ _ _ _ _ _ _ _ _ _ _ _ _ TRUE ("Priority Message? (F)") _] -> w15
      tunnel: w10 -> [_ w30 _ _ _ _ _ _ _ _ _ _ _ _ _]
      tunnel: w8 -> [w22 w39 w42 w62 w82 w97 w112 w139 w184 w230 w270 w312 w320 w343 w360]
      tunnel: "Used functions" -> [_ _ _ _ _ _ w121 w144 w190 w235 w278 _ _ w344 _]
      tunnel: [w22 w37 w42 w62 w82 w100 w114 w140 w185 w231 w269 w312 w320 w343 w360] -> w7
      frame Default {
        # "The Defualt Case run if there is a message that isn't defined in any of the other cases.\nOutput a program error"
        n7 = Format Into String(format string="The invalid message string \"%s\" was  received in the Parameter Analyzer Loop", w24) -> (resulting string=w26:string)  [unwired: 2 in, 1 out]
        n8 = call <vilib>:"Error Cluster From Error Code.vi"("error message (\"\")"=w26, "error code (0)"=5001) -> ("error out"=w23:errorcluster)  [unwired: 2 in, 5 out]
      }
      frame "Initialize" {
        n9 = Unbundle By Name(w40) -> ("Parameter Analyzer"=w34:refnum<queue>, "Message Handler Loop"=w31:refnum<queue>)
        n10 = call "Enqueue Message (Single).vi"("error in (no error)"=w36, "Message"="Parameter Analyzer - Update Refnums", "Message Queue"=w31) -> ("error out"=w33:errorcluster)  [unwired: 1 in, 7 out]
        n11 = call "Enqueue Message (Single).vi"("error in (no error)"=w33, "Message Data"=w30, "Message"="Parameter Analyzer - Set UI", "Message Queue"=w31) -> ("error out"=w29:errorcluster)  [unwired: 7 out]
        n12 = call "Enqueue Message (Single).vi"("error in (no error)"=w29, "Message"="Check if Refnum Update", "Message Queue"=w34) -> ("error out"=w28:errorcluster)  [unwired: 1 in, 7 out]
        n13 = Bundle By Name(cluster=w39, "Configuration"=w30) -> (w37:T58)
      }
      frame "Check if Refnum Update" {
        n14 = Unbundle By Name(w42) -> ("Initialization.Update Refnums"=w41:bool)
        n15 = case shown="False" w41 {
          tunnel: w45 -> [w50 w55]
          tunnel: [w47 w52] -> w44
          tunnel: w43 -> [w46 w51]
          frame True {
            n16 = Unbundle By Name(w50) -> ("Parameter Analyzer"=w48:refnum<queue>)
            n17 = call "Enqueue Message (Single).vi"("error in (no error)"=w46, "Message"="Continue Initialize", "Message Queue"=w48) -> ("error out"=w47:errorcluster)  [unwired: 1 in, 7 out]
          }
          frame False {
            n18 = Unbundle By Name(w55) -> ("Parameter Analyzer"=w53:refnum<queue>)
            n19 = call "Enqueue Message (Single).vi"("error in (no error)"=w51, "Message"="Check if Refnum Update", "Message Queue"=w53) -> ("error out"=w52:errorcluster)  [unwired: 1 in, 7 out]
          }
        }
      }
      frame "Continue Initialize" {
        n20 = Unbundle By Name(w58) -> ("Save Data.Ready"=w59:refnum<notifier>)
        n21 = Wait on Notification(notifier=w59, error in (no error)=w57) -> (error out=w56:errorcluster)  [unwired: 2 in, 3 out]
        n22 = Unbundle By Name(w62) -> ("Configuration"=w60:T2, "Configuration.Acquisition Mode"=w61:enum32{"Sweeping Mode", "Sampling Mode"})
        n23 = Unbundle By Name(w71) -> ("Parameter Analyzer"=w64:refnum<queue>)
        n24 = call "Enqueue Message (Single).vi"("error in (no error)"=w56, "Message Data"=w60, "Message"="Update Visa Session", "Message Queue"=w64) -> ("error out"=w72:errorcluster)  [unwired: 7 out]
        n25 = call "Enqueue Message (Single).vi"("error in (no error)"=w72, "Message Data"=w60, "Message"="Configure Integration Time", "Message Queue"=w64) -> ("error out"=w68:errorcluster)  [unwired: 7 out]
        n26 = case shown="\"Sweeping Mode\", Default" w61 {
          tunnel: ["Configure Sweeping" ("Message") "Configure Sampling" ("Message")] -> w67
          frame "Sweeping Mode", Default {
          }
          frame "Sampling Mode" {
          }
        }
        n27 = call "Enqueue Message (Single).vi"("error in (no error)"=w68, "Message Data"=w60, "Message"=w67, "Message Queue"=w64) -> ("error out"=w66:errorcluster)  [unwired: 7 out]
        n28 = call "Enqueue Message (Single).vi"("error in (no error)"=w66, "Message"="Ready", "Message Queue"=w64) -> ("error out"=w65:errorcluster)  [unwired: 1 in, 7 out]
      }
      frame "Ready" {
        n29 = Unbundle By Name(w82) -> ("Initialization.Update Visa Session"=w83:bool, "Initialization.Configure Integration Time"=w79:bool, "Initialization.Configure Acquisition Mode"=w80:bool, "Initialization.Update Refnums"=w81:bool)
        n30 = Compound Arithmetic op=AND(w83, w79, w80, w81) -> (w84:bool)
        n31 = case shown="True" w84 {
          tunnel: [w87 w92] -> w76
          tunnel: w78 -> [w86 w91]
          tunnel: w77 -> [w85 _]
          tunnel: w75 -> [_ w90]
          frame False {
            n32 = Unbundle By Name(w85) -> ("Parameter Analyzer"=w89:refnum<queue>)
            n33 = call "Enqueue Message (Single).vi"("error in (no error)"=w86, "Message"="Ready", "Message Queue"=w89) -> ("error out"=w87:errorcluster)  [unwired: 1 in, 7 out]
          }
          frame True {
            n34 = Unbundle By Name(w90) -> ("Parameter Analyzer.Ready"=w93:refnum<notifier>)
            n35 = Send Notification(notification=TRUE, notifier=w93, error in (no error)=w91) -> (error out=w92:errorcluster)  [unwired: 1 out]
          }
        }
      }
      frame "Update Refnums" {
        n36 = Unbundle By Name(w97) -> ("Refnums"=w96:T59)
        n37 = Variant To Data(error in=w107, type=w96, Variant=w109) -> (data=w95:T59, error out=w108:errorcluster)
        n38 = Unbundle By Name(w102) -> ("Parameter Analyzer"=w98:T46)
        n39 = Bundle By Name(cluster=w97, "Initialization.Update Refnums"=TRUE, "Refnums"=w95) -> (w100:T58)
        n40 = call "Parameter Analyzer.vi"("Function"=Parameter_Analyzer_Functions."Update Refnums", "HP4155C Refnums"=w95, "Error in"=w108, "Parameter Analyzer Notifiers"=w98) -> ("error out"=w105:errorcluster)  [unwired: 17 in, 6 out]
        n41 = call "Update Status.vi"("error in"=w105, "String"="Parameter Analyzer Refnums updated" ("button name (\"OK\")"), "Message Queues out"=w103) -> ("error out"=w106:errorcluster)  [unwired: 8 out]
      }
      frame "Update Visa Session" {
        n42 = Unbundle By Name(w112) -> ("Configuration"=w111:T2)
        n43 = Variant To Data(error in=w122, type=w111, Variant=w124) -> (data=w117:T2, error out=w123:errorcluster)
        n44 = Unbundle By Name(w117) -> ("Parameter Analyzer VISA Session"=w110:refnum<visa-resource-name>)
        n45 = case shown="True" w121 {
          tunnel: w123 -> [w128 w133]
          tunnel: [w127 w134] -> w116
          tunnel: w115 -> [w130 _]
          tunnel: w110 -> [_ w132]
          frame False {
            n46 = Unbundle By Name(w130) -> ("Parameter Analyzer.Status"=w129:refnum<notifier>)
            n47 = One Button Dialog(message="Parameter Analyzer VISA Session Updated" ("button name (\"OK\")")) -> ()  [unwired: 2 out]
            n48 = Send Notification(notification="Connected", notifier=w129, error in (no error)=w128) -> (error out=w127:errorcluster)  [unwired: 1 out]
          }
          frame True {
            n49 = call "Parameter Analyzer.vi"("Function"=Parameter_Analyzer_Functions."Connect", "VISA Session"=w132, "Error in"=w133) -> ("error out"=w134:errorcluster)  [unwired: 18 in, 6 out]
          }
        }
        n50 = Bundle By Name(cluster=w112, "Initialization.Update Visa Session"=TRUE, "Configuration.Parameter Analyzer VISA Session"=w110) -> (w114:T58)
        n51 = call "Update Status.vi"("error in"=w116, "String"="Parameter Analyzer VISA Session Updated" ("button name (\"OK\")"), "Message Queues out"=w119) -> ("error out"=w120:errorcluster)  [unwired: 8 out]
      }
      frame "Configure Sweeping" {
        n52 = Unbundle By Name(w139) -> ("Configuration"=w138:T2)
        n53 = Variant To Data(error in=w145, type=w138, Variant=w147) -> (data=w141:T2, error out=w146:errorcluster)
        n54 = case shown="True" w144 {
          tunnel: w146 -> [w154 w180]
          tunnel: [w149 w165] -> w137
          tunnel: w141 -> [_ w179]
          tunnel: w139 -> [w157 w178]
          tunnel: [w156 w163] -> w140
          tunnel: w136 -> [w148 _]
          tunnel: w135 -> [_ w164]
          frame False {
            n55 = call "Dialog.vi"("error in (no error)"=w154, "message"="Parameter Analyzer Sweeping Configuration Updated" ("button name (\"OK\")")) -> ("error out"=w150:errorcluster)  [unwired: 1 in, 8 out]
            n56 = Bundle By Name(cluster=w157, "Initialization.Configure Acquisition Mode"=TRUE ("Initialization.Configure Integration Time")) -> (w156:T58)
            n57 = Unbundle By Name(w148) -> ("Parameter Analyzer.Status"=w152:refnum<notifier>)
            n58 = Send Notification(notification="Sweeping Configured", notifier=w152, error in (no error)=w150) -> (error out=w149:errorcluster)  [unwired: 1 out]
          }
          frame True {
            w159 = TRUE ("Initialization.Configure Integration Time")
            n59 = Unbundle By Name(w179) -> ("SMU 1 - Sweeping"=w177:T4, "SMU 2 - Sweeping"=w176:T4, "SMU 3 - Sweeping"=w175:T4, "SMU 4 - Sweeping"=w174:T4, "Sweep Spacing"=w173:T5, "Range"=w172:T6, "Sweeping Time Parameters"=w160:T3)
            n60 = call "Parameter Analyzer.vi"("Function"=Parameter_Analyzer_Functions."Configure Sweeping", "Error in"=w180, "SMU 1 - Sweeping"=w177, "SMU 2 - Sweeping"=w176, "SMU 3 - Sweeping"=w175, "SMU 4 - Sweeping"=w174, "Sweep Spacing"=w173, "Range"=w172) -> ("error out"=w166:errorcluster)  [unwired: 13 in, 6 out]
            n61 = Bundle By Name(cluster=w178, "Initialization.Configure Integration Time"=w159, "Initialization.Configure Acquisition Mode"=w159, "Configuration.Acquisition Mode"=enum32{"Sweeping Mode", "Sampling Mode"}."Sweeping Mode", "Configuration.SMU 1 - Sweeping"=w177, "Configuration.SMU 2 - Sweeping"=w176, "Configuration.SMU 3 - Sweeping"=w175, "Configuration.SMU 4 - Sweeping"=w174, "Configuration.Sweep Spacing"=w173, "Configuration.Range"=w172, "Configuration.Sweeping Time Parameters"=w160) -> (w163:T58)
            n62 = Unbundle By Name(w163) -> ("Configuration"=w162:T2)
            n63 = call "Configuration to String.vi"("error in (no error)"=w166, "Configuration"=w162, "Instrument"=Instrument_List."Parameter Analyzer") -> ("error out"=w170:errorcluster, "Instrument Configuration"=w167:T33)  [unwired: 7 out]
            n64 = Unbundle By Name(w164) -> ("Save Data"=w171:refnum<queue>)
            n65 = call "Enqueue Message (Single).vi"("error in (no error)"=w170, "Message Data"=w167, "Message"="Set Instrument Configuration", "Message Queue"=w171) -> ("error out"=w165:errorcluster)  [unwired: 7 out]
          }
        }
        n66 = call "Update Status.vi"("error in"=w137, "String"="Parameter Analyzer Sweeping Configured" ("button name (\"OK\")"), "Message Queues out"=w135) -> ("error out"=w143:errorcluster)  [unwired: 8 out]
      }
      frame "Configure Sampling" {
        n67 = Unbundle By Name(w184) -> ("Configuration"=w183:T2)
        n68 = Variant To Data(error in=w191, type=w183, Variant=w193) -> (data=w186:T2, error out=w192:errorcluster)
        n69 = case shown="True" w190 {
          tunnel: w192 -> [w195 w225]
          tunnel: [w197 w209] -> w188
          tunnel: w186 -> [_ w224]
          tunnel: [w201 w210] -> w185
          tunnel: w184 -> [w202 w223]
          tunnel: w182 -> [w196 _]
          tunnel: w181 -> [_ w207]
          frame False {
            n70 = call "Dialog.vi"("error in (no error)"=w195, "message"="Parameter Analyzer Sampling Configuration Updated" ("button name (\"OK\")")) -> ("error out"=w194:errorcluster)  [unwired: 1 in, 8 out]
            n71 = Bundle By Name(cluster=w202, "Initialization.Configure Acquisition Mode"=TRUE ("Initialization.Configure Integration Time")) -> (w201:T58)
            n72 = Unbundle By Name(w196) -> ("Parameter Analyzer.Status"=w199:refnum<notifier>)
            n73 = Send Notification(notification="Sampling Configured", notifier=w199, error in (no error)=w194) -> (error out=w197:errorcluster)  [unwired: 1 out]
          }
          frame True {
            n74 = Unbundle By Name(w224) -> ("Range"=w215:T6, "SMU1 - Sampling"=w216:T7, "SMU2 - Sampling"=w217:T7, "SMU3 - Sampling"=w218:T7, "SMU4 - Sampling"=w219:T7, "Sampling Time Parameters"=w220:T8, "Stop Condition"=w221:T9)
            n75 = call "Parameter Analyzer.vi"("Function"=Parameter_Analyzer_Functions."Configure Sampling", "Error in"=w225, "SMU1 - Sampling"=w216, "SMU2 - Sampling"=w217, "SMU3 - Sampling"=w218, "SMU4 - Sampling"=w219, "Sampling Time Parameters"=w220, "Range"=w215, "Stop Condition"=w221) -> ("error out"=w209:errorcluster)  [unwired: 12 in, 6 out]
            n76 = Bundle By Name(cluster=w223, "Configuration.Acquisition Mode"=enum32{"Sweeping Mode", "Sampling Mode"}."Sampling Mode", "Initialization.Configure Acquisition Mode"=TRUE ("Initialization.Configure Integration Time"), "Configuration.Range"=w215, "Configuration.SMU1 - Sampling"=w216, "Configuration.SMU2 - Sampling"=w217, "Configuration.SMU3 - Sampling"=w218, "Configuration.SMU4 - Sampling"=w219, "Configuration.Sampling Time Parameters"=w220, "Configuration.Stop Condition"=w221) -> (w210:T58)
            n77 = Unbundle By Name(w210) -> ("Configuration"=w208:T2)
            n78 = call "Configuration to String.vi"("error in (no error)"=w209, "Configuration"=w208, "Instrument"=Instrument_List."Parameter Analyzer") -> ("error out"=w213:errorcluster, "Instrument Configuration"=w211:T33)  [unwired: 7 out]
            n79 = Unbundle By Name(w207) -> ("Save Data"=w214:refnum<queue>)
            n80 = call "Enqueue Message (Single).vi"("error in (no error)"=w213, "Message Data"=w211, "Message"="Set Instrument Configuration", "Message Queue"=w214) -> ()  [unwired: 8 out]
          }
        }
        n81 = call "Update Status.vi"("error in"=w188, "String"="Parameter Analyzer Sampling Configured" ("button name (\"OK\")"), "Message Queues out"=w181) -> ("error out"=w189:errorcluster)  [unwired: 8 out]
      }
      frame "Configure Integration Time" {
        n82 = Unbundle By Name(w230) -> ("Configuration"=w229:T2)
        n83 = Variant To Data(error in=w236, type=w229, Variant=w238) -> (data=w232:T2, error out=w237:errorcluster)
        n84 = case shown="True" w235 {
          tunnel: w237 -> [w242 w263]
          tunnel: [w240 w254] -> w228
          tunnel: w232 -> [_ w264]
          tunnel: w230 -> [w248 w262]
          tunnel: [w247 w252] -> w231
          tunnel: w227 -> [w239 _]
          tunnel: w226 -> [_ w257]
          frame False {
            n85 = call "Dialog.vi"("error in (no error)"=w242, "message"="Parameter Analyzer Integration Time Updated" ("button name (\"OK\")")) -> ("error out"=w241:errorcluster)  [unwired: 1 in, 8 out]
            n86 = Unbundle By Name(w239) -> ("Parameter Analyzer.Status"=w243:refnum<notifier>)
            n87 = Bundle By Name(cluster=w248, "Initialization.Configure Integration Time"=TRUE) -> (w247:T58)
            n88 = Send Notification(notification="Integration Time Configured", notifier=w243, error in (no error)=w241) -> (error out=w240:errorcluster)  [unwired: 1 out]
          }
          frame True {
            n89 = Unbundle By Name(w264) -> ("Sweeping Time Parameters"=w260:T3)
            n90 = Bundle By Name(cluster=w262, "Initialization.Configure Integration Time"=TRUE, "Configuration.Sweeping Time Parameters"=w260) -> (w252:T58)
            n91 = call "Parameter Analyzer.vi"("Function"=Parameter_Analyzer_Functions."Configure Integration Time", "User Integration Time"=w260, "Error in"=w263) -> ("error out"=w256:errorcluster)  [unwired: 18 in, 6 out]
            n92 = Unbundle By Name(w252) -> ("Configuration"=w251:T2)
            n93 = call "Configuration to String.vi"("error in (no error)"=w256, "Configuration"=w251, "Instrument"=Instrument_List."Parameter Analyzer") -> ("error out"=w255:errorcluster, "Instrument Configuration"=w253:T33)  [unwired: 7 out]
            n94 = Unbundle By Name(w257) -> ("Save Data"=w258:refnum<queue>)
            n95 = call "Enqueue Message (Single).vi"("error in (no error)"=w255, "Message Data"=w253, "Message"="Set Instrument Configuration", "Message Queue"=w258) -> ("error out"=w254:errorcluster)  [unwired: 7 out]
          }
        }
        n96 = call "Update Status.vi"("error in"=w228, "String"="Parameter Analyzer Integration Time  Configured" ("button name (\"OK\")"), "Message Queues out"=w226) -> ("error out"=w234:errorcluster)  [unwired: 8 out]
      }
      frame "Measure" {
        n97 = Unbundle By Name(w270) -> ("Configuration"=w271:T2)
        n98 = Variant To Data(error in=w273, type=w271, Variant=w266) -> (data=w268:T2, error out=w272:errorcluster)
        n99 = Unbundle By Name(w268) -> ("Status Polling Time (ms)"=w267:u32)
        n100 = case shown="True" w278 {
          tunnel: w272 -> [w281 w304]
          tunnel: [w292 w297] -> w275
          tunnel: w274 -> [w291 _]
          tunnel: w270 -> [w287 w301]
          tunnel: [w286 w303] -> w269
          tunnel: w267 -> [w285 w302]
          tunnel: w265 -> [_ w298]
          frame False {
            n101 = Unbundle By Name(w291) -> ("Parameter Analyzer.Measurement"=w290:refnum<notifier>, "Parameter Analyzer.Status"=w279:refnum<notifier>)
            n102 = Send Notification(notification="Measuring", notifier=w279, error in (no error)=w281) -> (error out=w280:errorcluster)  [unwired: 1 out]
            n103 = Bundle By Name(cluster=w287, "Configuration.Status Polling Time (ms)"=w285) -> (w286:T58)
            n104 = call "Dialog.vi"("error in (no error)"=w280, "message"="Parameter Analyzer Measuring") -> ("error out"=w284:errorcluster)  [unwired: 1 in, 8 out]
            n105 = Send Notification(notification=T63 {"Sequence"=[1.0, 2.0, 3.0, 4.0, 5.0, 6.0, 7.0, 8.0, 9.0, 10.0, 11.0, 12.0, 13.0, 14.0, 15.0, 16.0, 17.0, 18.0, 19.0, 20.0, 21.0, 22.0, 23.0, 24.0, 25.0, 26.0, 27.0, 28.0, 29.0, 30.0, 31.0, 32.0, 33.0, 34.0, 35.0, 36.0, 37.0, 38.0, 39.0, 40.0, 41.0, 42.0, 43.0, 44.0, 45.0, 46.0, 47.0, 48.0, 49.0, 50.0, 51.0, 52.0, 53.0, 54.0, 55.0, 56.0, 57.0, 58.0, 59.0, 60.0, 61.0, 62.0, 63.0, 64.0, 65.0, 66.0, 67.0, 68.0, 69.0, 70.0, 71.0, 72.0, 73.0, 74.0, 75.0, 76.0, 77.0, 78.0, 79.0, 80.0, 81.0, 82.0, 83.0, 84.0, 85.0, 86.0, 87.0, 88.0, 89.0, 90.0, 91.0, 92.0, 93.0, 94.0, 95.0, 96.0, 97.0, 98.0, 99.0, 100.0, 101.0], "V1"=[0.0, 0.01, 0.02, 0.030000000000000002, 0.04, 0.05, 0.060000000000000005, 0.07, 0.08, 0.09000000000000001, 0.1, 0.11, 0.12000000000000001, 0.13, 0.14, 0.15, 0.16, 0.17, 0.18000000000000002, 0.19, 0.2, 0.21000000000000002, 0.22, 0.23, 0.24000000000000002, 0.25, 0.26, 0.27, 0.28, 0.29000000000000004, 0.3, 0.31, 0.32, 0.33, 0.34, 0.35000000000000003, 0.36000000000000004, 0.37, 0.38, 0.39, 0.4, 0.41000000000000003, 0.42000000000000004, 0.43, 0.44, 0.45, 0.46, 0.47000000000000003, 0.48000000000000004, 0.49000000000000005, 0.5, 0.51, 0.52, 0.53, 0.54, 0.55, 0.56, 0.5700000000000001, 0.5800000000000001, 0.5900000000000001, 0.6, 0.61, 0.62, 0.63, 0.64, 0.65, 0.66, 0.67, 0.68, 0.6900000000000001, 0.7000000000000001, 0.7100000000000001, 0.7200000000000001, 0.73, 0.74, 0.75, 0.76, 0.77, 0.78, 0.79, 0.8, 0.81, 0.8200000000000001, 0.8300000000000001, 0.8400000000000001, 0.8500000000000001, 0.86, 0.87, 0.88, 0.89, 0.9, 0.91, 0.92, 0.93, 0.9400000000000001, 0.9500000000000001, 0.9600000000000001, 0.9700000000000001, 0.9800000000000001, 0.9900000000000001, 1.0], "V2"=[-0.00028, -0.00028, -0.00028, -0.00028, -0.00028, -0.00028, -0.00028, -0.00028, -0.00028, -0.00028, -0.00028, -0.00028, -0.0003, -0.0003, -0.0003, -0.0003, -0.0003, -0.0003, -0.0003, -0.0003, -0.0003, -0.0003, -0.0003, -0.0003, -0.00031999999999999997, -0.00031999999999999997, -0.00031999999999999997, -0.00031999999999999997, -0.00031999999999999997, -0.00031999999999999997, -0.00031999999999999997, -0.00031999999999999997, -0.00031999999999999997, -0.00031999999999999997, -0.00031999999999999997, -0.00031999999999999997, -0.00033999999999999997, -0.00033999999999999997, -0.00033999999999999997, -0.00033999999999999997, -0.00033999999999999997, -0.00033999999999999997, -0.00033999999999999997, -0.00033999999999999997, -0.00033999999999999997, -0.00033999999999999997, -0.00033999999999999997, -0.00035999999999999997, -0.00035999999999999997, -0.00035999999999999997, -0.00035999999999999997, -0.00035999999999999997, -0.00035999999999999997, -0.00035999999999999997, -0.00035999999999999997, -0.00035999999999999997, -0.00035999999999999997, -0.00035999999999999997, -0.00037999999999999997, -0.00037999999999999997, -0.00037999999999999997, -0.00037999999999999997, -0.00037999999999999997, -0.00037999999999999997, -0.00037999999999999997, -0.00037999999999999997, -0.00037999999999999997, -0.00037999999999999997, -0.00037999999999999997, -0.00039999999999999996, -0.00039999999999999996, -0.00039999999999999996, -0.00039999999999999996, -0.00039999999999999996, -0.00039999999999999996, -0.00039999999999999996, -0.00039999999999999996, -0.00039999999999999996, -0.00037999999999999997, -0.00037999999999999997, -0.00037999999999999997, -0.00037999999999999997, -0.00037999999999999997, -0.00037999999999999997, -0.00037999999999999997, -0.00037999999999999997, -0.00037999999999999997, -0.00037999999999999997, -0.00037999999999999997, -0.00035999999999999997, -0.00035999999999999997, -0.00035999999999999997, -0.00035999999999999997, -0.00035999999999999997, -0.00035999999999999997, -0.00035999999999999997, -0.00035999999999999997, -0.00035999999999999997, -0.00035999999999999997, -0.00035999999999999997, -0.00033999999999999997], "V3"=[-0.00028, -0.00028, -0.00028, -0.00028, -0.00028, -0.00028, -0.00028, -0.00028, -0.00028, -0.00028, -0.00028, -0.00028, -0.00028, -0.00028, -0.00028, -0.00028, -0.00028, -0.00028, -0.00028, -0.00028, -0.00028, -0.00028, -0.00028, -0.00028, -0.00028, -0.00028, -0.00028, -0.00028, -0.00028, -0.00028, -0.00028, -0.00028, -0.00028, -0.00028, -0.00028, -0.00028, -0.00028, -0.00028, -0.00028, -0.00028, -0.00028, -0.00028, -0.00028, -0.00028, -0.00028, -0.00028, -0.00028, -0.00028, -0.00028, -0.00028, -0.00028, -0.00028, -0.00028, -0.00028, -0.00028, -0.00028, -0.00028, -0.00028, -0.00028, -0.00028, -0.00028, -0.00028, -0.00028, -0.00028, -0.00028, -0.00028, -0.00028, -0.00028, -0.00028, -0.00028, -0.00028, -0.00028, -0.00028, -0.00028, -0.00028, -0.00028, -0.00028, -0.00028, -0.00028, -0.00028, -0.00028, -0.00028, -0.00028, -0.00028, -0.00028, -0.00028, -0.00028, -0.00028, -0.00028, -0.00028, -0.00028, -0.00028, -0.00028, -0.00028, -0.00028, -0.00028, -0.00028, -0.00028, -0.00028, -0.00028, -0.00028], "V4"=[0.0, 0.0, 0.0, 0.0, 0.0, 0.0, 0.0, 0.0, 0.0, 0.0, 0.0, 0.0, 0.0, 0.0, 0.0, 0.0, 0.0, 0.0, 0.0, 0.0, 0.0, 0.0, 0.0, 0.0, 0.0, 0.0, 0.0, 0.0, 0.0, 0.0, 0.0, 0.0, 0.0, 0.0, 0.0, 0.0, 0.0, 0.0, 0.0, 0.0, 0.0, 0.0, 0.0, 0.0, 0.0, 0.0, 0.0, 0.0, 0.0, 0.0, 0.0, 0.0, 0.0, 0.0, 0.0, 0.0, 0.0, 0.0, 0.0, 0.0, 0.0, 0.0, 0.0, 0.0, 0.0, 0.0, 0.0, 0.0, 0.0, 0.0, 0.0, 0.0, 0.0, 0.0, 0.0, 0.0, 0.0, 0.0, 0.0, 0.0, 0.0, 0.0, 0.0, 0.0, 0.0, 0.0, 0.0, 0.0, 0.0, 0.0, 0.0, 0.0, 0.0, 0.0, 0.0, 0.0, 0.0, 0.0, 0.0, 0.0, 0.0], "I1"=[1.4e-13, 1.3e-13, 1.2e-13, 1.3e-13, 1.2e-13, 1.4e-13, 1.1e-13, 1.5e-13, 1.2e-13, 1.5e-13, 1e-13, 1.2e-13, 1.3e-13, 1e-13, 1.2e-13, 1.4e-13, 1.1e-13, 1.2e-13, 1.4e-13, 1.1e-13, 1.1e-13, 1.3e-13, 1e-13, 1.1e-13, 1.3e-13, 1e-13, 1.1e-13, 1.3e-13, 1e-13, 1.1e-13, 1.2e-13, 1.1e-13, 1e-13, 1.1e-13, 1.1e-13, 1e-13, 1.1e-13, 1.1e-13, 9.000000000000001e-14, 1.1e-13, 1.1e-13, 9.000000000000001e-14, 1e-13, 1.2e-13, 9.000000000000001e-14, 1e-13, 1.2e-13, 9.000000000000001e-14, 1e-13, 1.2e-13, 9.000000000000001e-14, 1e-13, 1.2e-13, 9.000000000000001e-14, 1e-13, 1.1e-13, 9.000000000000001e-14, 9.000000000000001e-14, 1.1e-13, 8e-14, 9.000000000000001e-14, 1e-13, 9.000000000000001e-14, 9.000000000000001e-14, 9.000000000000001e-14, 9.000000000000001e-14, 8e-14, 9.000000000000001e-14, 9.000000000000001e-14, 8e-14, 9.000000000000001e-14, 9.000000000000001e-14, 7e-14, 9.000000000000001e-14, 9.000000000000001e-14, 7e-14, 8e-14, 9.000000000000001e-14, 7e-14, 8e-14, 9.000000000000001e-14, 7e-14, 8e-14, 9.000000000000001e-14, 7e-14, 8e-14, 9.000000000000001e-14, 7e-14, 7e-14, 9.000000000000001e-14, 7e-14, 7e-14, 9.000000000000001e-14, 6.000000000000001e-14, 7e-14, 9.000000000000001e-14, 6.000000000000001e-14, 7e-14, 8e-14, 6.000000000000001e-14, 7e-14], "I2"=[0.0, 0.0, 0.0, 0.0, 0.0, 0.0, 0.0, 0.0, 0.0, 0.0, 0.0, 0.0, 0.0, 0.0, 0.0, 0.0, 0.0, 0.0, 0.0, 0.0, 0.0, 0.0, 0.0, 0.0, 0.0, 0.0, 0.0, 0.0, 0.0, 0.0, 0.0, 0.0, 0.0, 0.0, 0.0, 0.0, 0.0, 0.0, 0.0, 0.0, 0.0, 0.0, 0.0, 0.0, 0.0, 0.0, 0.0, 0.0, 0.0, 0.0, 0.0, 0.0, 0.0, 0.0, 0.0, 0.0, 0.0, 0.0, 0.0, 0.0, 0.0, 0.0, 0.0, 0.0, 0.0, 0.0, 0.0, 0.0, 0.0, 0.0, 0.0, 0.0, 0.0, 0.0, 0.0, 0.0, 0.0, 0.0, 0.0, 0.0, 0.0, 0.0, 0.0, 0.0, 0.0, 0.0, 0.0, 0.0, 0.0, 0.0, 0.0, 0.0, 0.0, 0.0, 0.0, 0.0, 0.0, 0.0, 0.0, 0.0, 0.0], "I3"=[0.0, 0.0, 0.0, 0.0, 0.0, 0.0, 0.0, 0.0, 0.0, 0.0, 0.0, 0.0, 0.0, 0.0, 0.0, 0.0, 0.0, 0.0, 0.0, 0.0, 0.0, 0.0, 0.0, 0.0, 0.0, 0.0, 0.0, 0.0, 0.0, 0.0, 0.0, 0.0, 0.0, 0.0, 0.0, 0.0, 0.0, 0.0, 0.0, 0.0, 0.0, 0.0, 0.0, 0.0, 0.0, 0.0, 0.0, 0.0, 0.0, 0.0, 0.0, 0.0, 0.0, 0.0, 0.0, 0.0, 0.0, 0.0, 0.0, 0.0, 0.0, 0.0, 0.0, 0.0, 0.0, 0.0, 0.0, 0.0, 0.0, 0.0, 0.0, 0.0, 0.0, 0.0, 0.0, 0.0, 0.0, 0.0, 0.0, 0.0, 0.0, 0.0, 0.0, 0.0, 0.0, 0.0, 0.0, 0.0, 0.0, 0.0, 0.0, 0.0, 0.0, 0.0, 0.0, 0.0, 0.0, 0.0, 0.0, 0.0, 0.0], "I4"=[1.6e-13, 1.3e-13, 1.5e-13, 1.3e-13, 1.4e-13, 1.4e-13, 1.3e-13, 1.4e-13, 1.2e-13, 1.4e-13, 1.5e-13, 1.2e-13, 1.4e-13, 1.5e-13, 1.2e-13, 1.4e-13, 1.6e-13, 1.3e-13, 1.4e-13, 1.7e-13, 1.3e-13, 1.4e-13, 1.7e-13, 1.3e-13, 1.4e-13, 1.7e-13, 1.3e-13, 1.5e-13, 1.7e-13, 1.3e-13, 1.5e-13, 1.6e-13, 1.4e-13, 1.5e-13, 1.6e-13, 1.5e-13, 1.4e-13, 1.6e-13, 1.5e-13, 1.4e-13, 1.6e-13, 1.6e-13, 1.4e-13, 1.6e-13, 1.7e-13, 1.4e-13, 1.6e-13, 1.8e-13, 1.4e-13, 1.6e-13, 1.9e-13, 1.5e-13, 1.6e-13, 1.9e-13, 1.5e-13, 1.7e-13, 2e-13, 1.6e-13, 1.7e-13, 2e-13, 1.6e-13, 1.7e-13, 1.9e-13, 1.6e-13, 1.7e-13, 1.9e-13, 1.7e-13, 1.7e-13, 1.8e-13, 1.7e-13, 1.7e-13, 1.8e-13, 1.8e-13, 1.7e-13, 1.8e-13, 1.9e-13, 1.6e-13, 1.9e-13, 2e-13, 1.6e-13, 1.9e-13, 1.9e-13, 1.6e-13, 1.9e-13, 1.9e-13, 1.7e-13, 1.9e-13, 1.8e-13, 1.8e-13, 2e-13, 1.8e-13, 1.9e-13, 2e-13, 1.7e-13, 1.9e-13, 2e-13, 1.7e-13, 1.9e-13, 1.9e-13, 1.7e-13, 2e-13]} ("Measurement"), notifier=w290, error in (no error)=w284) -> (error out=w288:errorcluster)  [unwired: 1 out]
            n106 = Send Notification(notification="Measurement Performed", notifier=w279, error in (no error)=w288) -> (error out=w292:errorcluster)  [unwired: 1 out]
          }
          frame True {
            n107 = Bundle By Name(cluster=w301, "Configuration.Status Polling Time (ms)"=w302) -> (w303:T58)
            n108 = call "Parameter Analyzer.vi"("Function"=Parameter_Analyzer_Functions."Measure", "Status Polling Time (ms)"=w302, "Error in"=w304) -> ("Electrical Measurement"=w295:T39, "error out"=w296:errorcluster)  [unwired: 18 in, 5 out]
            n109 = Unbundle By Name(w298) -> ("Save Data"=w299:refnum<queue>)
            n110 = call "Enqueue Message (Single).vi"("error in (no error)"=w296, "Message Data"=w295, "Message"="Set Electrical Measurement", "Message Queue"=w299) -> ("error out"=w297:errorcluster)  [unwired: 7 out]
          }
        }
        n111 = call "Update Status.vi"("error in"=w275, "String"="Parameter Analyzer  Measurement Performed" ("button name (\"OK\")"), "Message Queues out"=w265) -> ("error out"=w276:errorcluster)  [unwired: 8 out]
      }
      frame "Save Electrical Measurement" {
        n112 = call "Set Device Information.vi"() -> ("error out"=w306:errorcluster, "Workspace Info"=w305:T32, "OK?"=w308:bool)  [unwired: 1 in, 8 out]
        n113 = Merge Errors(w306, w310) -> (w307:errorcluster)
        n114 = case shown="True" w308 {
          tunnel: w311 -> [_ w317]
          tunnel: w307 -> [w313 w316]
          tunnel: [w313 w315] -> w309
          tunnel: w305 -> [_ w314]
          frame False {
          }
          frame True {
            n115 = Unbundle By Name(w317) -> ("Save Data"=w318:refnum<queue>)
            n116 = call "Enqueue Message (Single).vi"("error in (no error)"=w316, "Message Data"=w314, "Message"="Save Electrical Measurement", "Message Queue"=w318) -> ("error out"=w315:errorcluster)  [unwired: 7 out]
          }
        }
      }
      frame "Error" {
        # "Clear Errors to avoid getting stuck \nin repeating this case"
        # "Add here Cases that are handled \nalready by the Message Handler Loop"
        n117 = Variant To Data(error in=w328, type=errorcluster {"status"=FALSE, "code"=0, "source"=""} ("error out"), Variant=w321) -> (data=w327:errorcluster, error out=w326:errorcluster)
        n118 = Merge Errors(w327, w326) -> (w325:errorcluster)
        n119 = Unbundle By Name(w329) -> ("Message Handler Loop"=w331:refnum<queue>)
        n120 = Unbundle By Name(w325) -> ("code"=w322:i32)
        n121 = case shown="Default" w322 {
          tunnel: w331 -> [w335]
          tunnel: w325 -> [w333]
          tunnel: [w332] -> w324
          frame Default {
            n122 = call "Enqueue Message (Single).vi"("Message Data"=w333, "Message"="Error", "Message Queue"=w335) -> ("error out"=w332:errorcluster)  [unwired: 1 in, 7 out]
          }
        }
        n123 = call <vilib>:"Clear Errors.vi"("error in (no error)"=w324) -> ("error out"=w323:errorcluster)  [unwired: 1 in, 5 out]
      }
      frame "Exit" {
        w340 = TRUE ("Priority Message? (F)")
        # "Stip the VI"
        n124 = case shown="True" w344 {
          tunnel: w346 -> [w352 w358]
          tunnel: [w351 w359] -> w345
          tunnel: w338 -> [w350 _]
          frame False {
            n125 = Unbundle By Name(w350) -> ("Parameter Analyzer.Status"=w353:refnum<notifier>)
            n126 = Send Notification(notification="Disconnected", notifier=w353, error in (no error)=w352) -> (error out=w351:errorcluster)  [unwired: 1 out]
          }
          frame True {
            n127 = call "Wait.vi"("error in (no error)"=w358, "milliseconds to wait"=u32 50) -> ("error out"=w357:errorcluster)  [unwired: 9 in]
            n128 = call "Parameter Analyzer.vi"("Function"=Parameter_Analyzer_Functions."Disconnect", "Error in"=w357) -> ("error out"=w359:errorcluster)  [unwired: 19 in, 6 out]
          }
        }
        n129 = Unbundle By Name(w348) -> ("Parameter Analyzer"=w349:refnum<queue>)
        n130 = Unbundle By Name(w338) -> ("Parameter Analyzer.Exit"=w339:refnum<notifier>, "Parameter Analyzer.Ready"=w342:refnum<notifier>)
        n131 = Release Queue(queue=w349, error in (no error)=w345) -> (error out=w337:errorcluster)  [unwired: 3 out]
        n132 = Send Notification(notification=w340, notifier=w342, error in (no error)=w337) -> (error out=w341:errorcluster)  [unwired: 1 out]
        n133 = Send Notification(notification=w340, notifier=w339, error in (no error)=w341) -> (error out=w336:errorcluster)  [unwired: 1 out]
      }
      frame "Notify Status" {
        n134 = Unbundle By Name(w362) -> ("Parameter Analyzer.Instrument Data"=w361:refnum<notifier>)
        n135 = Send Notification(notification=w360, notifier=w361, error in (no error)=w364) -> (error out=w363:errorcluster)  [unwired: 1 out]
      }
    }
    n136 = call "Message Handling Loop.vi"("error in (no error)"=w14, "Message Queue"=w12) -> ("dup error in"=w13:errorcluster)  [unwired: 9 out]
  }
  "error out" <- w2
